vi "Motors 2.vi"(1 "Cluster":T1, 2 "Motors Visa Ref":refnum<visa-resource-name>="COM7") -> ()   [LabVIEW 2010]
panel:
  in  "Steps to deactivate hard limit after finding datums":dbl=500.0
  out "Loop i":i32
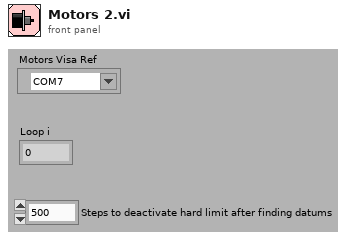
[diagram p1: front panel]
types:
  T1 = cluster{"Stop X?":refnum<vi>, "Stop Y?":refnum<vi>, "Stop Z?":refnum<vi>, "Stop Theta?":refnum<vi>, "Backlash?":refnum<vi>, "Backlash X":refnum<vi>, "Backlash Y":refnum<vi>, "Backlash Z":refnum<vi>, "Backlash Theta":refnum<vi>, "Manual IO?":refnum<vi>, "Manual Communication is Active\n(Close Before Ending Program)":refnum<vi>, "Reset Motors?":refnum<vi>, "Set Jogger?":refnum<vi>, "Normal":refnum<vi>, "Fast":refnum<vi>, "Jogger Axis":refnum<vi>, "Redefine Origin as Current Location?":refnum<vi>, "Save Current Motor Parameters?":refnum<vi>, "Find Datums Nearest Hard Limits?":refnum<vi>, "Saved Limits":refnum<vi>, "Use Datums Nearest Hard Limits to Reset Origin?":refnum<vi>, "X Go?":refnum<vi>, "Y Go?":refnum<vi>, "Z Go?":refnum<vi>, "Theta Go?":refnum<vi>, "Jog-Mode":refnum<vi>, "x+?":refnum<vi>, "x-?":refnum<vi>, "y+?":refnum<vi>, "y-?":refnum<vi>, "z+?":refnum<vi>, "z-?":refnum<vi>, "theta+?":refnum<vi>, "theta-?":refnum<vi>, "X Set Slew Speed?":refnum<vi>, "(mm/s)":refnum<vi>, "Y Set Slew Speed?":refnum<vi>, "(mm/s)":refnum<vi>, "Z Set Slew Speed?":refnum<vi>, "(mm/s)":refnum<vi>, "Theta Set Slew Speed?":refnum<vi>, "(degrees/s)":refnum<vi>, "Go To Saved Position?":refnum<vi>, "Defined Positions":refnum<vi>, "Need to Update Motor Parameters":refnum<vi>, "X Jogger Normal Speed":refnum<vi>, "X Jogger Fast Speed":refnum<vi>, "Y Jogger Normal Speed":refnum<vi>, "Y Jogger Fast Speed":refnum<vi>, "Z Jogger Normal Speed":refnum<vi>, "Z Jogger Fast Speed":refnum<vi>, "Theta Jogger Normal Speed":refnum<vi>, "Theta Jogger Fast Speed":refnum<vi>, "X Moving":refnum<vi>, "Y Moving":refnum<vi>, "Z Moving":refnum<vi>, "Theta Moving":refnum<vi>, "X Slew Speed (mm or degree/s)":refnum<vi>, "Y Slew Speed (mm or degree/s)":refnum<vi>, "Z Slew Speed (mm or degree/s)":refnum<vi>, "Theta Slew Speed (mm or degree/s)":refnum<vi>, "X-Axis (mm)":refnum<vi>, "Y-Axis (mm)":refnum<vi>, "Z-Axis (mm)":refnum<vi>, "Theta (deg)":refnum<vi>, "X Multiplier":refnum<vi>, "Y Multiplier":refnum<vi>, "Z Multiplier":refnum<vi>, "Theta Multiplier":refnum<vi>, "Motors Online":refnum<vi>, "Motors Status":refnum<vi>, "Status X":refnum<vi>, "Status Y":refnum<vi>, "Status Z":refnum<vi>, "Status Theta":refnum<vi>, "Motors error":refnum<vi>, "QUIT":refnum<vi>, "EMERGENCY":refnum<vi>, "X Go To":refnum<vi>, "Y Go To":refnum<vi>, "Z Go To":refnum<vi>, "Theta Go To":refnum<vi>, "Delta X (mm)":refnum<vi>, "Delta Y (mm)":refnum<vi>, "Delta Z (mm)":refnum<vi>, "Delta Theta (deg)":refnum<vi>, "X Speed (mm/s)":refnum<vi>, "Y Speed (mm/s)":refnum<vi>, "Z Speed (mm/s)":refnum<vi>, "Theta Speed (deg/s)":refnum<vi>, "x+":refnum<vi>, "x-":refnum<vi>, "y+":refnum<vi>, "y-":refnum<vi>, "z+":refnum<vi>, "z-":refnum<vi>, "theta+":refnum<vi>, "theta-":refnum<vi>, "Saved Positions":refnum<vi>}
  T2 = cluster{"X Set Slew Speed?":refnum<vi>, "(mm/s)":refnum<vi>, "Y Set Slew Speed?":refnum<vi>, "(mm/s)":refnum<vi>, "Z Set Slew Speed?":refnum<vi>, "(mm/s)":refnum<vi>, "Theta Set Slew Speed?":refnum<vi>, "(degrees/s)":refnum<vi>, "Need to Update Motor Parameters":refnum<vi>, "X Multiplier":refnum<vi>, "Y Multiplier":refnum<vi>, "Z Multiplier":refnum<vi>, "Theta Multiplier":refnum<vi>}
  T3 = cluster{"Jog-Mode":refnum<vi>, "y+?":refnum<vi>, "y-?":refnum<vi>, "Y Moving":refnum<vi>, "Delta Y (mm)":refnum<vi>, "Y Multiplier":refnum<vi>, "y+":refnum<vi>, "y-":refnum<vi>, "Y-Axis (mm)":refnum<vi>, "Status Y":refnum<vi>, "Y Speed (mm/s)":refnum<vi>}
  T4 = cluster{"Jog-Mode":refnum<vi>, "z+?":refnum<vi>, "z-?":refnum<vi>, "Z Speed (mm/s)":refnum<vi>, "Delta Z (mm)":refnum<vi>, "Z Multiplier":refnum<vi>, "Z-Axis (mm)":refnum<vi>, "Status Z":refnum<vi>, "z+":refnum<vi>, "z-":refnum<vi>, "Z Moving":refnum<vi>}
  T5 = cluster{"Jog-Mode":refnum<vi>, "theta+?":refnum<vi>, "theta-?":refnum<vi>, "Theta Speed (deg/s)":refnum<vi>, "Delta Theta (deg)":refnum<vi>, "Theta Multiplier":refnum<vi>, "Theta (deg)":refnum<vi>, "Status Theta":refnum<vi>, "theta+":refnum<vi>, "theta-":refnum<vi>, "Theta Moving":refnum<vi>}
  T6 = cluster{"Stop X?":refnum<vi>, "Stop Y?":refnum<vi>, "Stop Z?":refnum<vi>, "Stop Theta?":refnum<vi>}
  T7 = cluster{"Backlash?":refnum<vi>, "Backlash X":refnum<vi>, "Backlash Y":refnum<vi>, "Backlash Z":refnum<vi>, "Backlash Theta":refnum<vi>}
  T8 = cluster{"EMERGENCY":refnum<vi>, "Manual IO?":refnum<vi>, "Manual Communication is Active\n(Close Before Ending Program)":refnum<vi>, "Reset Motors?":refnum<vi>}
  T9 = cluster{"Redefine Origin as Current Location?":refnum<vi>, "Save Current Motor Parameters?":refnum<vi>}
  T10 = cluster{"Set Jogger?":refnum<vi>, "Normal":refnum<vi>, "Fast":refnum<vi>, "Jogger Axis":refnum<vi>, "X Multiplier":refnum<vi>, "Y Multiplier":refnum<vi>, "Z Multiplier":refnum<vi>, "Theta Multiplier":refnum<vi>, "Need to Update Motor Parameters":refnum<vi>}
  T11 = cluster{"Find Datums Nearest Hard Limits?":refnum<vi>, "X Multiplier":refnum<vi>, "Y Multiplier":refnum<vi>, "Z Multiplier":refnum<vi>, "Theta Multiplier":refnum<vi>, "X-Axis (mm)":refnum<vi>, "Y-Axis (mm)":refnum<vi>, "Z-Axis (mm)":refnum<vi>, "Theta (deg)":refnum<vi>, "Status X":refnum<vi>, "Status Y":refnum<vi>, "Status Z":refnum<vi>, "Status Theta":refnum<vi>, "X Moving":refnum<vi>, "Y Moving":refnum<vi>, "Z Moving":refnum<vi>, "Theta Moving":refnum<vi>, "Saved Limits":refnum<vi>}
  T12 = cluster{"Use Datums Nearest Hard Limits to Reset Origin?":refnum<vi>, "X Multiplier":refnum<vi>, "Y Multiplier":refnum<vi>, "Z Multiplier":refnum<vi>, "Theta Multiplier":refnum<vi>, "X-Axis (mm)":refnum<vi>, "Y-Axis (mm)":refnum<vi>, "Z-Axis (mm)":refnum<vi>, "Theta (deg)":refnum<vi>, "Status X":refnum<vi>, "Status Y":refnum<vi>, "Status Z":refnum<vi>, "Status Theta":refnum<vi>}
  T13 = cluster{"X Go?":refnum<vi>, "X Multiplier":refnum<vi>, "X Go To":refnum<vi>, "Y Go?":refnum<vi>, "Y Multiplier":refnum<vi>, "Y Go To":refnum<vi>, "Z Go?":refnum<vi>, "Z Multiplier":refnum<vi>, "Z Go To":refnum<vi>, "Theta Go?":refnum<vi>, "Theta Multiplier":refnum<vi>, "Theta Go To":refnum<vi>}
  T14 = cluster{"Jog-Mode":refnum<vi>, "x+?":refnum<vi>, "x-?":refnum<vi>, "X Moving":refnum<vi>, "X Multiplier":refnum<vi>, "Delta X (mm)":refnum<vi>, "X Speed (mm/s)":refnum<vi>, "x+":refnum<vi>, "x-":refnum<vi>, "X-Axis (mm)":refnum<vi>, "Status X":refnum<vi>}
  T15 = cluster{"Go To Saved Position?":refnum<vi>, "Defined Positions":refnum<vi>, "X Multiplier":refnum<vi>, "Y Multiplier":refnum<vi>, "Z Multiplier":refnum<vi>, "Theta Multiplier":refnum<vi>, void}
  T16 = cluster{"Status X":refnum<vi>, "X-Axis (mm)":refnum<vi>, "X Multiplier":refnum<vi>, "X Moving":refnum<vi>, "Status Y":refnum<vi>, "Y-Axis (mm)":refnum<vi>, "Y Multiplier":refnum<vi>, "Y Moving":refnum<vi>, "Status Z":refnum<vi>, "Z-Axis (mm)":refnum<vi>, "Z Multiplier":refnum<vi>, "Z Moving":refnum<vi>, "Status Theta":refnum<vi>, "Theta (deg)":refnum<vi>, "Theta Multiplier":refnum<vi>, "Theta Moving":refnum<vi>}
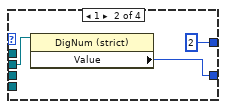
[diagram p3: hidden frame]
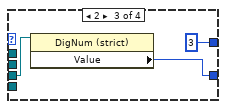
[diagram p4: hidden frame]
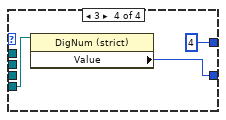
[diagram p5: hidden frame]
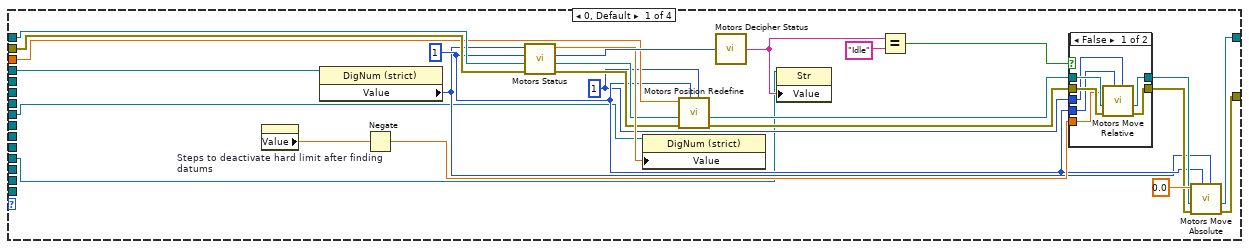
[diagram p15: hidden frame]
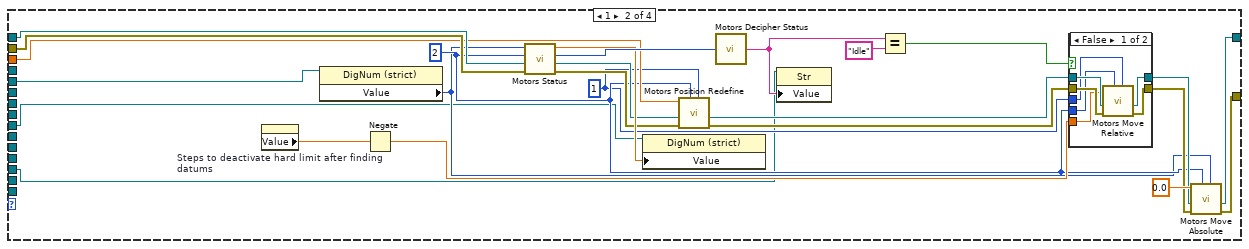
[diagram p17: hidden frame]
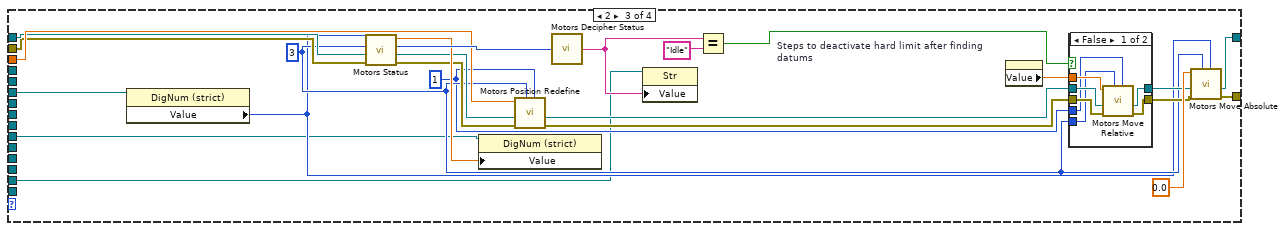
[diagram p19: hidden frame]
diagram:
  n1 = Unbundle("Cluster") -> ("Stop X?"=w101:refnum<vi>, "Stop Y?"=w100:refnum<vi>, "Stop Z?"=w99:refnum<vi>, "Stop Theta?"=w98:refnum<vi>, "Backlash?"=w97:refnum<vi>, "Backlash X"=w96:refnum<vi>, "Backlash Y"=w95:refnum<vi>, "Backlash Z"=w94:refnum<vi>, "Backlash Theta"=w93:refnum<vi>, "Manual IO?"=w91:refnum<vi>, "Manual Communication is Active\n(Close Before Ending Program)"=w90:refnum<vi>, "Reset Motors?"=w89:refnum<vi>, "Set Jogger?"=w85:refnum<vi>, "Normal"=w84:refnum<vi>, "Fast"=w83:refnum<vi>, "Jogger Axis"=w82:refnum<vi>, "Redefine Origin as Current Location?"=w80:refnum<vi>, "Save Current Motor Parameters?"=w79:refnum<vi>, "Find Datums Nearest Hard Limits?"=w77:refnum<vi>, "Saved Limits"=w71:refnum<vi>, "Use Datums Nearest Hard Limits to Reset Origin?"=w72:refnum<vi>, "X Go?"=w69:refnum<vi>, "Y Go?"=w67:refnum<vi>, "Z Go?"=w65:refnum<vi>, "Theta Go?"=w63:refnum<vi>, "Jog-Mode"=w41:refnum<vi>, "x+?"=w60:refnum<vi>, "x-?"=w59:refnum<vi>, "y+?"=w53:refnum<vi>, "y-?"=w52:refnum<vi>, "z+?"=w47:refnum<vi>, "z-?"=w46:refnum<vi>, "theta+?"=w40:refnum<vi>, "theta-?"=w39:refnum<vi>, "X Set Slew Speed?"=w31:refnum<vi>, "(mm/s)"=w30:refnum<vi>, "Y Set Slew Speed?"=w29:refnum<vi>, "(mm/s)"=w28:refnum<vi>, "Z Set Slew Speed?"=w27:refnum<vi>, "(mm/s)"=w26:refnum<vi>, "Theta Set Slew Speed?"=w25:refnum<vi>, "(degrees/s)"=w24:refnum<vi>, "Go To Saved Position?"=w8:refnum<vi>, "Defined Positions"=w7:refnum<vi>, "Need to Update Motor Parameters"=w23:refnum<vi>, "X Moving"=w13:refnum<vi>, "Y Moving"=w12:refnum<vi>, "Z Moving"=w11:refnum<vi>, "Theta Moving"=w10:refnum<vi>, "X-Axis (mm)"=w17:refnum<vi>, "Y-Axis (mm)"=w16:refnum<vi>, "Z-Axis (mm)"=w15:refnum<vi>, "Theta (deg)"=w14:refnum<vi>, "X Multiplier"=w6:refnum<vi>, "Y Multiplier"=w4:refnum<vi>, "Z Multiplier"=w3:refnum<vi>, "Theta Multiplier"=w5:refnum<vi>, "Motors Online"=w73:refnum<vi>, "Motors Status"=w76:refnum<vi>, "Status X"=w21:refnum<vi>, "Status Y"=w20:refnum<vi>, "Status Z"=w19:refnum<vi>, "Status Theta"=w18:refnum<vi>, "Motors error"=w74:refnum<vi>, "QUIT"=w105:refnum<vi>, "EMERGENCY"=w88:refnum<vi>, "X Go To"=w68:refnum<vi>, "Y Go To"=w66:refnum<vi>, "Z Go To"=w64:refnum<vi>, "Theta Go To"=w62:refnum<vi>, "Delta X (mm)"=w58:refnum<vi>, "Delta Y (mm)"=w51:refnum<vi>, "Delta Z (mm)"=w44:refnum<vi>, "Delta Theta (deg)"=w37:refnum<vi>, "X Speed (mm/s)"=w57:refnum<vi>, "Y Speed (mm/s)"=w48:refnum<vi>, "Z Speed (mm/s)"=w45:refnum<vi>, "Theta Speed (deg/s)"=w38:refnum<vi>, "x+"=w56:refnum<vi>, "x-"=w55:refnum<vi>, "y+"=w50:refnum<vi>, "y-"=w49:refnum<vi>, "z+"=w43:refnum<vi>, "z-"=w42:refnum<vi>, "theta+"=w36:refnum<vi>, "theta-"=w35:refnum<vi>)  [unwired: 13 out]
  n2 = Bundle("X Set Slew Speed?"=w31, "(mm/s)"=w30, "Y Set Slew Speed?"=w29, "(mm/s)"=w28, "Z Set Slew Speed?"=w27, "(mm/s)"=w26, "Theta Set Slew Speed?"=w25, "(degrees/s)"=w24, "Need to Update Motor Parameters"=w23, "X Multiplier"=w6, "Y Multiplier"=w4, "Z Multiplier"=w3, "Theta Multiplier"=w5) -> (w22:T2)  [unwired: 1 in]
  n3 = Bundle("Jog-Mode"=w41, "y+?"=w53, "y-?"=w52, "Y Moving"=w12, "Delta Y (mm)"=w51, "Y Multiplier"=w4, "y+"=w50, "y-"=w49, "Y-Axis (mm)"=w16, "Status Y"=w20, "Y Speed (mm/s)"=w48) -> (w34:T3)  [unwired: 1 in]
  n4 = Bundle("Jog-Mode"=w41, "z+?"=w47, "z-?"=w46, "Z Speed (mm/s)"=w45, "Delta Z (mm)"=w44, "Z Multiplier"=w3, "Z-Axis (mm)"=w15, "Status Z"=w19, "z+"=w43, "z-"=w42, "Z Moving"=w11) -> (w33:T4)  [unwired: 1 in]
  n5 = Bundle("Jog-Mode"=w41, "theta+?"=w40, "theta-?"=w39, "Theta Speed (deg/s)"=w38, "Delta Theta (deg)"=w37, "Theta Multiplier"=w5, "Theta (deg)"=w14, "Status Theta"=w18, "theta+"=w36, "theta-"=w35, "Theta Moving"=w10) -> (w32:T5)  [unwired: 1 in]
  n6 = Bundle("Stop X?"=w101, "Stop Y?"=w100, "Stop Z?"=w99, "Stop Theta?"=w98) -> (w87:T6)  [unwired: 1 in]
  n7 = Bundle("Backlash?"=w97, "Backlash X"=w96, "Backlash Y"=w95, "Backlash Z"=w94, "Backlash Theta"=w93) -> (w92:T7)  [unwired: 1 in]
  n8 = Bundle("EMERGENCY"=w88, "Manual IO?"=w91, "Manual Communication is Active\n(Close Before Ending Program)"=w90, "Reset Motors?"=w89) -> (w86:T8)  [unwired: 1 in]
  n9 = Bundle("Redefine Origin as Current Location?"=w80, "Save Current Motor Parameters?"=w79) -> (w78:T9)  [unwired: 1 in]
  n10 = Bundle("Set Jogger?"=w85, "Normal"=w84, "Fast"=w83, "Jogger Axis"=w82, "X Multiplier"=w6, "Y Multiplier"=w4, "Z Multiplier"=w3, "Theta Multiplier"=w5, "Need to Update Motor Parameters"=w23) -> (w81:T10)  [unwired: 1 in]
  n11 = Bundle("Find Datums Nearest Hard Limits?"=w77, "X Multiplier"=w6, "Y Multiplier"=w4, "Z Multiplier"=w3, "Theta Multiplier"=w5, "X-Axis (mm)"=w17, "Y-Axis (mm)"=w16, "Z-Axis (mm)"=w15, "Theta (deg)"=w14, "Status X"=w21, "Status Y"=w20, "Status Z"=w19, "Status Theta"=w18, "X Moving"=w13, "Y Moving"=w12, "Z Moving"=w11, "Theta Moving"=w10, "Saved Limits"=w71) -> (w75:T11)  [unwired: 1 in]
  n12 = Bundle("Use Datums Nearest Hard Limits to Reset Origin?"=w72, "X Multiplier"=w6, "Y Multiplier"=w4, "Z Multiplier"=w3, "Theta Multiplier"=w5, "X-Axis (mm)"=w17, "Y-Axis (mm)"=w16, "Z-Axis (mm)"=w15, "Theta (deg)"=w14, "Status X"=w21, "Status Y"=w20, "Status Z"=w19, "Status Theta"=w18) -> (w70:T12)  [unwired: 1 in]
  n13 = Bundle("X Go?"=w69, "X Multiplier"=w6, "X Go To"=w68, "Y Go?"=w67, "Y Multiplier"=w4, "Y Go To"=w66, "Z Go?"=w65, "Z Multiplier"=w3, "Z Go To"=w64, "Theta Go?"=w63, "Theta Multiplier"=w5, "Theta Go To"=w62) -> (w61:T13)  [unwired: 1 in]
  n14 = Bundle("Jog-Mode"=w41, "x+?"=w60, "x-?"=w59, "X Moving"=w13, "X Multiplier"=w6, "Delta X (mm)"=w58, "X Speed (mm/s)"=w57, "x+"=w56, "x-"=w55, "X-Axis (mm)"=w17, "Status X"=w21) -> (w54:T14)  [unwired: 1 in]
  n15 = property on="Property Node" class="Str"(reference=w76, "Value"="Opening Communications") -> (reference out=w104:refnum<vi>)  [unwired: 1 in, 1 out]
  n16 = call "Motors Open.vi"("VISA in"="Motors Visa Ref") -> ("error out"=w109:errorcluster, "VISA out"=w106:refnum<visa-resource-name>)  [unwired: 1 in]
  n17 = property on="Property Node" class="Bool (strict)"(reference=w23, "Value"=TRUE) -> ()  [unwired: 1 in, 2 out]
  n18 = call <vilib>:"Simple Error Handler.vi"("error in (no error)"=w109) -> ("error?"=w108:bool, "error out"=w110:errorcluster)  [unwired: 4 in, 3 out]
  n19 = property on="Property Node" class="Clust (strict)"(reference=w74, "Value"=w110) -> ()  [unwired: 1 in, 2 out]
  n20 = Bundle("Go To Saved Position?"=w8, "Defined Positions"=w7, "X Multiplier"=w6, "Y Multiplier"=w4, "Z Multiplier"=w3, "Theta Multiplier"=w5) -> (w2:T15)  [unwired: 2 in]
  n21 = Bundle("Status X"=w21, "X-Axis (mm)"=w17, "X Multiplier"=w6, "X Moving"=w13, "Status Y"=w20, "Y-Axis (mm)"=w16, "Y Multiplier"=w4, "Y Moving"=w12, "Status Z"=w19, "Z-Axis (mm)"=w15, "Z Multiplier"=w3, "Z Moving"=w11, "Status Theta"=w18, "Theta (deg)"=w14, "Theta Multiplier"=w5, "Theta Moving"=w10) -> (w9:T16)  [unwired: 1 in]
  n22 = Not(x=w108) -> (.not. x?=w107:bool)
  n23 = case shown="True" w107 {
    tunnel: w104 -> [_ w131]
    tunnel: w106 -> [_ w130]
    tunnel: w74 -> [_ w129]
    tunnel: w105 -> [_ w128]
    tunnel: w92 -> [_ w126]
    tunnel: w87 -> [_ w125]
    tunnel: w86 -> [_ w124]
    tunnel: w81 -> [_ w123]
    tunnel: w78 -> [_ w122]
    tunnel: w75 -> [_ w121]
    tunnel: w70 -> [_ w120]
    tunnel: w61 -> [_ w119]
    tunnel: w54 -> [_ w118]
    tunnel: w34 -> [_ w117]
    tunnel: w33 -> [_ w116]
    tunnel: w32 -> [_ w115]
    tunnel: w22 -> [_ w114]
    tunnel: w9 -> [_ w113]
    tunnel: w2 -> [_ w112]
    frame False {
    }
    frame True {
      n24 = property on="Property Node" class="Str"(reference=w131, "Value"="Running") -> (reference out=w127:refnum<vi>)  [unwired: 1 in, 1 out]
      n25 = while {
        shift-right: _ -> [_]
        shift-left: w130 -> [w324]
        tunnel: w129 -> [w421]
        tunnel: w128 -> [w368]
        tunnel: w127 -> [w365]
        tunnel: w126 -> [w313]
        tunnel: w125 -> [w325]
        tunnel: w124 -> [w302]
        tunnel: w123 -> [w284]
        tunnel: w122 -> [w283]
        tunnel: w121 -> [w278]
        tunnel: w120 -> [w259]
        tunnel: w119 -> [w245]
        tunnel: w118 -> [w232]
        tunnel: w117 -> [w218]
        tunnel: w116 -> [w203]
        tunnel: w115 -> [w190]
        tunnel: w114 -> [w176]
        tunnel: w113 -> [w154]
        tunnel: w112 -> [w137]
        i -> [w369]
        stop <- w422 stop-if-true
        # "This loop contains all of the code that has to communicate directly with the manipulator motor controllers.  They are arranged linearly to ensure multiple serial I/O's are never attempted simultaneously.  Note that this loop executes very slowly (each serial I/O takes about 1/20 sec)."
        n26 = Unbundle(w325) -> ("Stop X?"=w340:refnum<vi>, "Stop Y?"=w341:refnum<vi>, "Stop Z?"=w342:refnum<vi>, "Stop Theta?"=w343:refnum<vi>)
        n27 = property on="Property Node" class="Bool (strict)"(reference=w340) -> (reference out=w339:refnum<vi>, "Value"=w332:bool)  [unwired: 1 in, 1 out]
        n28 = property on="Property Node" class="Clust (strict)"(reference=w421) -> ("Value"=w323:errorcluster)  [unwired: 1 in, 2 out]
        n29 = case shown="True" w332 {
          tunnel: w323 -> [w528 w536]
          tunnel: w324 -> [w529 w535]
          tunnel: [w529 w533] -> w331
          tunnel: [w528 w532] -> w330
          tunnel: w339 -> [_ w530]
          frame False {
          }
          frame True {
            n30 = property on="Property Node" class="Bool (strict)"(reference=w530, "Value"=FALSE) -> ()  [unwired: 1 in, 2 out]
            n31 = call "Motors Stop.vi"("error in"=w536, "Axis"=1, "VISA in"=w535) -> ("error out"=w532:errorcluster, "VISA out"=w533:refnum<visa-resource-name>)
          }
        }
        n32 = property on="Property Node" class="Bool (strict)"(reference=w341) -> (reference out=w338:refnum<vi>, "Value"=w333:bool)  [unwired: 1 in, 1 out]
        n33 = case shown="True" w333 {
          tunnel: w330 -> [w519 w527]
          tunnel: w331 -> [w520 w526]
          tunnel: [w520 w524] -> w329
          tunnel: [w519 w523] -> w328
          tunnel: w338 -> [_ w521]
          frame False {
          }
          frame True {
            n34 = property on="Property Node" class="Bool (strict)"(reference=w521, "Value"=FALSE) -> ()  [unwired: 1 in, 2 out]
            n35 = call "Motors Stop.vi"("error in"=w527, "Axis"=2, "VISA in"=w526) -> ("error out"=w523:errorcluster, "VISA out"=w524:refnum<visa-resource-name>)
          }
        }
        n36 = property on="Property Node" class="Bool (strict)"(reference=w342) -> (reference out=w337:refnum<vi>, "Value"=w334:bool)  [unwired: 1 in, 1 out]
        n37 = case shown="True" w334 {
          tunnel: w328 -> [w510 w518]
          tunnel: w329 -> [w511 w517]
          tunnel: [w511 w515] -> w327
          tunnel: [w510 w514] -> w326
          tunnel: w337 -> [_ w512]
          frame False {
          }
          frame True {
            n38 = property on="Property Node" class="Bool (strict)"(reference=w512, "Value"=FALSE) -> ()  [unwired: 1 in, 2 out]
            n39 = call "Motors Stop.vi"("error in"=w518, "Axis"=3, "VISA in"=w517) -> ("error out"=w514:errorcluster, "VISA out"=w515:refnum<visa-resource-name>)
          }
        }
        n40 = property on="Property Node" class="Bool (strict)"(reference=w343) -> (reference out=w336:refnum<vi>, "Value"=w335:bool)  [unwired: 1 in, 1 out]
        n41 = case shown="True" w335 {
          tunnel: w326 -> [w501 w509]
          tunnel: w327 -> [w502 w508]
          tunnel: [w502 w506] -> w314
          tunnel: [w501 w505] -> w315
          tunnel: w336 -> [_ w503]
          frame False {
          }
          frame True {
            n42 = property on="Property Node" class="Bool (strict)"(reference=w503, "Value"=FALSE) -> ()  [unwired: 1 in, 2 out]
            n43 = call "Motors Stop.vi"("error in"=w509, "Axis"=4, "VISA in"=w508) -> ("error out"=w505:errorcluster, "VISA out"=w506:refnum<visa-resource-name>)
          }
        }
        n44 = Unbundle(w313) -> ("Backlash?"=w320:refnum<vi>, "Backlash X"=w316:refnum<vi>, "Backlash Y"=w317:refnum<vi>, "Backlash Z"=w318:refnum<vi>, "Backlash Theta"=w319:refnum<vi>)
        n45 = property on="Property Node" class="Bool (strict)"(reference=w320) -> (reference out=w322:refnum<vi>, "Value"=w321:bool)  [unwired: 1 in, 1 out]
        n46 = case shown="True" w321 {
          tunnel: [w486 w500] -> w301
          tunnel: w316 -> [_ w499]
          tunnel: w317 -> [_ w497]
          tunnel: w318 -> [_ w495]
          tunnel: w319 -> [_ w493]
          tunnel: w322 -> [_ w490]
          tunnel: w314 -> [w486 w489]
          tunnel: w315 -> [w485 w488]
          tunnel: [w485 w487] -> w300
          frame False {
          }
          frame True {
            n47 = property on="Property Node" class="Bool (strict)"(reference=w490, "Value"=FALSE) -> ()  [unwired: 1 in, 2 out]
            n48 = property on="Property Node" class="DigNum (strict)"(reference=w499) -> ("Value"=w498:u32)  [unwired: 1 in, 2 out]
            n49 = property on="Property Node" class="DigNum (strict)"(reference=w497) -> ("Value"=w496:u32)  [unwired: 1 in, 2 out]
            n50 = property on="Property Node" class="DigNum (strict)"(reference=w495) -> ("Value"=w494:u32)  [unwired: 1 in, 2 out]
            n51 = property on="Property Node" class="DigNum (strict)"(reference=w493) -> ("Value"=w492:u32)  [unwired: 1 in, 2 out]
            n52 = call "Motors Backlash.vi"("X"=w498, "Y"=w496, "VISA in"=w489, "error in"=w488, "Z"=w494, "Theta"=w492) -> ("VISA out"=w500:refnum<visa-resource-name>, "error out"=w487:errorcluster)  [unwired: 2 in]
          }
        }
        n53 = Unbundle(w302) -> ("EMERGENCY"=w305:refnum<vi>, "Manual IO?"=w308:refnum<vi>, "Manual Communication is Active\n(Close Before Ending Program)"=w306:refnum<vi>, "Reset Motors?"=w310:refnum<vi>)
        n54 = property on="Property Node" class="Bool (strict)"(reference=w308) -> (reference out=w309:refnum<vi>, "Value"=w307:bool)  [unwired: 1 in, 1 out]
        n55 = case shown="True" w307 {
          tunnel: [w458 w471] -> w304
          tunnel: [w459 w461] -> w303
          tunnel: w305 -> [_ w468]
          tunnel: w306 -> [_ w467]
          tunnel: w309 -> [_ w463]
          tunnel: w301 -> [w459 w462]
          tunnel: w300 -> [w458 w460]
          frame False {
          }
          frame True {
            n56 = property on="Property Node" class="Bool (strict)"(reference=w463, "Value"=FALSE) -> ()  [unwired: 1 in, 2 out]
            n57 = flat-sequence {
              tunnel: w467 -> [w473]
              tunnel: [w472] -> w465
              tunnel: [w480] -> w470
              tunnel: [w479] -> w469
              tunnel: w468 -> [w478]
              tunnel: [w477] -> w466
              tunnel: w465 -> [w477]
              tunnel: w462 -> [w476]
              tunnel: w460 -> [w475]
              tunnel: [w483] -> w461
              tunnel: [w484] -> w471
              tunnel: w470 -> [w484]
              tunnel: w469 -> [w483]
              tunnel: w466 -> [w481]
              frame #0 {
                n58 = property on="Property Node" class="Bool (strict)"(reference=w473, "Value"=TRUE ("Manual Communication is Active\n(Close Before Ending Program) 2")) -> (reference out=w472:refnum<vi>)  [unwired: 1 in, 1 out]
              }
              frame #1 {
                n59 = call "Motors Manual IO.vi"("error in"=w475, "Emergency Stop Reference"=w478, "VISA in"=w476) -> ("error out"=w480:errorcluster, "VISA out"=w479:refnum<visa-resource-name>)
              }
              frame #2 {
                n60 = property on="Property Node" class="Bool (strict)"(reference=w481, "Value"=FALSE ("Manual Communication is Active\n(Close Before Ending Program)")) -> ()  [unwired: 1 in, 2 out]
              }
            }
          }
        }
        n61 = Unbundle(w284) -> ("Set Jogger?"=w287:refnum<vi>, "Normal"=w289:refnum<vi>, "Fast"=w290:refnum<vi>, "Jogger Axis"=w293:refnum<vi>, "X Multiplier"=w295:refnum<vi>, "Y Multiplier"=w296:refnum<vi>, "Z Multiplier"=w297:refnum<vi>, "Theta Multiplier"=w298:refnum<vi>, "Need to Update Motor Parameters"=w299:refnum<vi>)
        n62 = property on="Property Node" class="Ring (strict)"(reference=w293) -> ("Value"=w294:u16)  [unwired: 1 in, 2 out]
        n63 = property on="Property Node" class="Bool (strict)"(reference=w310) -> (reference out=w312:refnum<vi>, "Value"=w311:bool)  [unwired: 1 in, 1 out]
        n64 = case shown="0, Default" w294 {
          tunnel: [u32 1 u32 2 u32 3 u32 4] -> _
          tunnel: [w424 w427 w430 w433] -> w292
          tunnel: w295 -> [w423 _ _ _]
          tunnel: w296 -> [_ w426 _ _]
          tunnel: w298 -> [_ _ _ w432]
          tunnel: w297 -> [_ _ w429 _]
          frame 0, Default {
            n65 = property on="Property Node" class="DigNum (strict)"(reference=w423) -> ("Value"=w424:u32)  [unwired: 1 in, 2 out]
          }
          frame 1 {
            n66 = property on="Property Node" class="DigNum (strict)"(reference=w426) -> ("Value"=w427:u32)  [unwired: 1 in, 2 out]
          }
          frame 2 {
            n67 = property on="Property Node" class="DigNum (strict)"(reference=w429) -> ("Value"=w430:u32)  [unwired: 1 in, 2 out]
          }
          frame 3 {
            n68 = property on="Property Node" class="DigNum (strict)"(reference=w432) -> ("Value"=w433:u32)  [unwired: 1 in, 2 out]
          }
        }
        n69 = case shown="True" w311 {
          tunnel: [w450 w457] -> w285
          tunnel: [w451 w456] -> w286
          tunnel: w303 -> [w451 w455]
          tunnel: w304 -> [w450 w454]
          tunnel: w312 -> [_ w452]
          frame False {
          }
          frame True {
            n70 = property on="Property Node" class="Bool (strict)"(reference=w452, "Value"=FALSE) -> ()  [unwired: 1 in, 2 out]
            n71 = call "Motors Reset.vi"("error in"=w454, "VISA in"=w455) -> ("error out"=w457:errorcluster, "VISA out"=w456:refnum<visa-resource-name>)
          }
        }
        n72 = property on="Property Node" class="Bool (strict)"(reference=w287) -> (reference out=w291:refnum<vi>, "Value"=w288:bool)  [unwired: 1 in, 1 out]
        n73 = case shown="True" w288 {
          tunnel: [w436 w449] -> w280
          tunnel: [w435 w447] -> w281
          tunnel: w292 -> [_ w448]
          tunnel: w291 -> [_ w445]
          tunnel: w289 -> [_ w441]
          tunnel: w290 -> [_ w440]
          tunnel: w285 -> [w436 w439]
          tunnel: w286 -> [w435 w438]
          tunnel: w299 -> [_ w437]
          frame False {
          }
          frame True {
            n74 = property on="Property Node" class="Bool (strict)"(reference=w445, "Value"=FALSE ("Need to Update Motor Parameters")) -> ()  [unwired: 1 in, 2 out]
            n75 = property on="Property Node" class="Bool (strict)"(reference=w437, "Value"=TRUE) -> ()  [unwired: 1 in, 2 out]
            n76 = property on="Property Node" class="DigNum (strict)"(reference=w441) -> ("Value"=w444:dbl)  [unwired: 1 in, 2 out]
            n77 = property on="Property Node" class="DigNum (strict)"(reference=w440) -> ("Value"=w443:dbl)  [unwired: 1 in, 2 out]
            n78 = call "Motors Jogger Speed.vi"("Axis Multiplier"=w448, "error in"=w439, "VISA in"=w438, "Fast Speed (mm or degree/sec)"=w443, "Normal Speed (mm or degree/sec)"=w444) -> ("error out"=w449:errorcluster, "VISA out"=w447:refnum<visa-resource-name>)  [unwired: 5 in]
          }
        }
        n79 = Unbundle(w283) -> ("Redefine Origin as Current Location?"=w282:refnum<vi>, "Save Current Motor Parameters?"=w279:refnum<vi>)
        n80 = property on="Property Node" class="Bool (strict)"(reference=w279) -> (reference out=w357:refnum<vi>, "Value"=w356:bool)  [unwired: 1 in, 1 out]
        n81 = property on="Property Node" class="Bool (strict)"(reference=w282) -> (reference out=w355:refnum<vi>, "Value"=w367:bool)  [unwired: 1 in, 1 out]
        n82 = case shown="True" w367 {
          tunnel: w281 -> [w1662 w1669]
          tunnel: w280 -> [w1663 w1665]
          tunnel: [w1663 w1667] -> w358
          tunnel: [w1662 w1668] -> w420
          tunnel: w355 -> [_ w1664]
          frame False {
          }
          frame True {
            n83 = property on="Property Node" class="Bool (strict)"(reference=w1664, "Value"=FALSE) -> ()  [unwired: 1 in, 2 out]
            n84 = call "Motors Redefine Origin.vi"("error in"=w1665, "VISA in"=w1669) -> ("error out"=w1667:errorcluster, "VISA out"=w1668:refnum<visa-resource-name>)
          }
        }
        n85 = case shown="True" w356 {
          tunnel: w358 -> [w1655 w1661]
          tunnel: [w1655 w1660] -> w375
          tunnel: w420 -> [w1654 w1659]
          tunnel: [w1654 w1658] -> w374
          tunnel: w357 -> [_ w1657]
          frame False {
          }
          frame True {
            n86 = property on="Property Node" class="Bool (strict)"(reference=w1657, "Value"=FALSE) -> ()  [unwired: 1 in, 2 out]
            n87 = call "Motors Save.vi"("error in"=w1661, "VISA in"=w1659) -> ("error out"=w1660:errorcluster, "VISA out"=w1658:refnum<visa-resource-name>)
          }
        }
        n88 = property on="Property Node" class="Bool (strict)"(reference=w368) -> ("Value"=w422:bool)  [unwired: 1 in, 2 out]
        n89 = Unbundle(w278) -> ("Find Datums Nearest Hard Limits?"=w277:refnum<vi>, "X Multiplier"=w276:refnum<vi>, "Y Multiplier"=w275:refnum<vi>, "Z Multiplier"=w274:refnum<vi>, "Theta Multiplier"=w273:refnum<vi>, "X-Axis (mm)"=w272:refnum<vi>, "Y-Axis (mm)"=w271:refnum<vi>, "Z-Axis (mm)"=w270:refnum<vi>, "Theta (deg)"=w269:refnum<vi>, "Status X"=w268:refnum<vi>, "Status Y"=w267:refnum<vi>, "Status Z"=w266:refnum<vi>, "Status Theta"=w265:refnum<vi>, "X Moving"=w264:refnum<vi>, "Y Moving"=w263:refnum<vi>, "Z Moving"=w262:refnum<vi>, "Theta Moving"=w261:refnum<vi>, "Saved Limits"=w260:refnum<vi>)
        n90 = property on="Property Node" class="Bool (strict)"(reference=w277) -> (reference out=w360:refnum<vi>, "Value"=w366:bool)  [unwired: 1 in, 1 out]
        n91 = case shown="True" w366 {
          tunnel: w375 -> [w754 w785]
          tunnel: [w754 w783] -> w372
          tunnel: [w753 w784] -> w370
          tunnel: w374 -> [w753 w786]
          tunnel: w365 -> [w752 w778]
          tunnel: [w751 w775] -> w363
          tunnel: [w752 w774] -> w362
          tunnel: w360 -> [_ w773]
          tunnel: w276 -> [_ w771]
          tunnel: w275 -> [_ w770]
          tunnel: w274 -> [_ w769]
          tunnel: w273 -> [_ w768]
          tunnel: w272 -> [_ w767]
          tunnel: w271 -> [_ w766]
          tunnel: w270 -> [_ w765]
          tunnel: w269 -> [_ w764]
          tunnel: w268 -> [_ w763]
          tunnel: w267 -> [_ w762]
          tunnel: w266 -> [_ w761]
          tunnel: w265 -> [_ w760]
          tunnel: w264 -> [_ w759]
          tunnel: w263 -> [_ w758]
          tunnel: w262 -> [_ w757]
          tunnel: w261 -> [_ w756]
          tunnel: w260 -> [w751 w755]
          frame False {
          }
          frame True {
            n92 = property on="Property Node" class="Bool (strict)"(reference=w773, "Value"=FALSE) -> ()  [unwired: 1 in, 2 out]
            n93 = flat-sequence {
              tunnel: w785 -> [w791]
              tunnel: w786 -> [w792]
              tunnel: [w792] -> w782
              tunnel: [w791] -> w781
              tunnel: w778 -> [w788]
              tunnel: [w787] -> w776
              tunnel: w782 -> [w828]
              tunnel: w781 -> [w827]
              tunnel: [w823] -> w780
              tunnel: [w822] -> w779
              tunnel: [w812] -> w777
              tunnel: w776 -> [w812]
              tunnel: [w810] -> w775
              tunnel: w771 -> [w809]
              tunnel: w770 -> [w808]
              tunnel: w769 -> [w807]
              tunnel: w768 -> [w806]
              tunnel: w767 -> [w805]
              tunnel: w766 -> [w804]
              tunnel: w765 -> [w803]
              tunnel: w764 -> [w802]
              tunnel: w763 -> [w801]
              tunnel: w762 -> [w800]
              tunnel: w761 -> [w799]
              tunnel: w760 -> [w798]
              tunnel: w759 -> [w797]
              tunnel: w758 -> [w796]
              tunnel: w757 -> [w795]
              tunnel: w756 -> [w794]
              tunnel: w755 -> [w793]
              tunnel: [w938] -> w783
              tunnel: [w939] -> w784
              tunnel: w780 -> [w939]
              tunnel: w779 -> [w938]
              tunnel: w777 -> [w936]
              tunnel: [w935] -> w774
              frame #0 {
                n94 = call <vilib>:"Set Busy.vi"("disable click? (T)"=FALSE) -> ()  [unwired: 9 in, 2 out]
                n95 = property on="Property Node" class="Str"(reference=w788, "Value"="Finding Datums Nearest Hard Limits\nThis May Take a Few Minutes" ("Status")) -> (reference out=w787:refnum<vi>)  [unwired: 1 in, 1 out]
              }
              frame #1 {
                n96 = call "Motors Find Datums.vi"("error in"=w827, "VISA in"=w828) -> ("error out"=w824:errorcluster, "VISA out"=w825:refnum<visa-resource-name>)
                n97 = for {
                  N: 4 -> [_]
                  shift-right: [w848] -> w822
                  shift-left: w824 -> [w849]
                  shift-right: [w847] -> w823
                  shift-left: w825 -> [w850]
                  tunnel: [w846] -> w814 mode=indexing
                  tunnel: w809 -> [w844]
                  tunnel: w808 -> [w843]
                  tunnel: w807 -> [w842]
                  tunnel: w806 -> [w841]
                  tunnel: w805 -> [w840]
                  tunnel: w804 -> [w839]
                  tunnel: w803 -> [w838]
                  tunnel: w802 -> [w837]
                  tunnel: w801 -> [w836]
                  tunnel: w800 -> [w835]
                  tunnel: w799 -> [w834]
                  tunnel: w798 -> [w833]
                  tunnel: w797 -> [w832]
                  tunnel: w796 -> [w831]
                  tunnel: w795 -> [w830]
                  tunnel: w794 -> [w829]
                  i -> [w845]
                  n98 = case shown="0, Default" w845 {
                    tunnel: w849 -> [w863 w884 w905 w926]
                    tunnel: w850 -> [w864 w885 w906 w927]
                    tunnel: [w857 w878 w898 w919] -> w848
                    tunnel: [w858 w879 w899 w920] -> w847
                    tunnel: [w855 w876 w902 w923] -> w846
                    tunnel: w844 -> [w854 _ _ _]
                    tunnel: w843 -> [_ w875 _ _]
                    tunnel: w842 -> [_ _ w896 _]
                    tunnel: w841 -> [_ _ _ w917]
                    tunnel: w840 -> [w853 _ _ _]
                    tunnel: w839 -> [_ w874 _ _]
                    tunnel: w838 -> [_ _ w895 _]
                    tunnel: w837 -> [_ _ _ w916]
                    tunnel: w836 -> [w852 _ _ _]
                    tunnel: w835 -> [_ w873 _ _]
                    tunnel: w834 -> [_ _ w894 _]
                    tunnel: w833 -> [_ _ _ w915]
                    tunnel: w832 -> [w851 _ _ _]
                    tunnel: w831 -> [_ w872 _ _]
                    tunnel: w830 -> [_ _ w893 _]
                    tunnel: w829 -> [_ _ _ w914]
                    frame 0, Default {
                      w856 = 1 ("Axis")
                      n99 = property on="Property Node" class="DigNum (strict)"(reference=w854) -> ("Value"=w862:u32)  [unwired: 1 in, 2 out]
                      n100 = call "Motors Status.vi"("error in"=w863, "VISA in"=w864, "Axis"=w856, "Axis Multiplier"=w862) -> ("error out"=w859:errorcluster, "VISA out"=w860:refnum<visa-resource-name>, "OS"=w869:i32, "Actual Position (mm or deg)"=w861:dbl)  [unwired: 3 in]
                      n101 = property on="Property Node" class="DigNum (strict)"(reference=w853, "Value"=w861) -> ()  [unwired: 1 in, 2 out]
                      n102 = call "Motors Datum Position.vi"("error in"=w859, "VISA in"=w860, "Axis"=w856) -> ("error out"=w857:errorcluster, "VISA out"=w858:refnum<visa-resource-name>, "Datum Position (steps)"=w855:string)  [unwired: 5 in]
                      n103 = call "Motors Decipher Status.vi"("OS"=w869) -> ("Status"=w868:string)
                      n104 = property on="Property Node" class="Str"(reference=w852, "Value"=w868) -> ()  [unwired: 1 in, 2 out]
                      n105 = Equal?(x=w868, y="Idle") -> (x = y?=w866:bool)
                      n106 = case shown="False" w866 {
                        tunnel: [TRUE FALSE] -> w865
                        frame False {
                        }
                        frame True {
                        }
                      }
                      n107 = property on="Property Node" class="Bool (strict)"(reference=w851, "Value"=w865) -> ()  [unwired: 1 in, 2 out]
                    }
                    frame 1 {
                      w877 = 2 ("Axis")
                      n108 = property on="Property Node" class="DigNum (strict)"(reference=w875) -> ("Value"=w883:u32)  [unwired: 1 in, 2 out]
                      n109 = call "Motors Status.vi"("error in"=w884, "VISA in"=w885, "Axis"=w877, "Axis Multiplier"=w883) -> ("error out"=w880:errorcluster, "VISA out"=w881:refnum<visa-resource-name>, "OS"=w890:i32, "Actual Position (mm or deg)"=w882:dbl)  [unwired: 3 in]
                      n110 = property on="Property Node" class="DigNum (strict)"(reference=w874, "Value"=w882) -> ()  [unwired: 1 in, 2 out]
                      n111 = call "Motors Datum Position.vi"("error in"=w880, "VISA in"=w881, "Axis"=w877) -> ("error out"=w878:errorcluster, "VISA out"=w879:refnum<visa-resource-name>, "Datum Position (steps)"=w876:string)  [unwired: 5 in]
                      n112 = call "Motors Decipher Status.vi"("OS"=w890) -> ("Status"=w888:string)
                      n113 = property on="Property Node" class="Str"(reference=w873, "Value"=w888) -> ()  [unwired: 1 in, 2 out]
                      n114 = Equal?(x=w888, y="Idle") -> (x = y?=w887:bool)
                      n115 = case shown="False" w887 {
                        tunnel: [TRUE FALSE] -> w886
                        frame False {
                        }
                        frame True {
                        }
                      }
                      n116 = property on="Property Node" class="Bool (strict)"(reference=w872, "Value"=w886) -> ()  [unwired: 1 in, 2 out]
                    }
                    frame 2 {
                      w897 = 3 ("Axis")
                      n117 = property on="Property Node" class="DigNum (strict)"(reference=w896) -> ("Value"=w904:u32)  [unwired: 1 in, 2 out]
                      n118 = call "Motors Status.vi"("error in"=w905, "VISA in"=w906, "Axis"=w897, "Axis Multiplier"=w904) -> ("error out"=w900:errorcluster, "VISA out"=w901:refnum<visa-resource-name>, "OS"=w911:i32, "Actual Position (mm or deg)"=w903:dbl)  [unwired: 3 in]
                      n119 = property on="Property Node" class="DigNum (strict)"(reference=w895, "Value"=w903) -> ()  [unwired: 1 in, 2 out]
                      n120 = call "Motors Datum Position.vi"("error in"=w900, "VISA in"=w901, "Axis"=w897) -> ("error out"=w898:errorcluster, "VISA out"=w899:refnum<visa-resource-name>, "Datum Position (steps)"=w902:string)  [unwired: 5 in]
                      n121 = call "Motors Decipher Status.vi"("OS"=w911) -> ("Status"=w909:string)
                      n122 = property on="Property Node" class="Str"(reference=w894, "Value"=w909) -> ()  [unwired: 1 in, 2 out]
                      n123 = Equal?(x=w909, y="Idle") -> (x = y?=w908:bool)
                      n124 = case shown="False" w908 {
                        tunnel: [TRUE FALSE] -> w907
                        frame False {
                        }
                        frame True {
                        }
                      }
                      n125 = property on="Property Node" class="Bool (strict)"(reference=w893, "Value"=w907) -> ()  [unwired: 1 in, 2 out]
                    }
                    frame 3 {
                      w918 = 4 ("Axis")
                      n126 = property on="Property Node" class="DigNum (strict)"(reference=w917) -> ("Value"=w925:u32)  [unwired: 1 in, 2 out]
                      n127 = call "Motors Status.vi"("error in"=w926, "VISA in"=w927, "Axis"=w918, "Axis Multiplier"=w925) -> ("error out"=w921:errorcluster, "VISA out"=w922:refnum<visa-resource-name>, "OS"=w932:i32, "Actual Position (mm or deg)"=w924:dbl)  [unwired: 3 in]
                      n128 = property on="Property Node" class="DigNum (strict)"(reference=w916, "Value"=w924) -> ()  [unwired: 1 in, 2 out]
                      n129 = call "Motors Datum Position.vi"("error in"=w921, "VISA in"=w922, "Axis"=w918) -> ("error out"=w919:errorcluster, "VISA out"=w920:refnum<visa-resource-name>, "Datum Position (steps)"=w923:string)  [unwired: 5 in]
                      n130 = call "Motors Decipher Status.vi"("OS"=w932) -> ("Status"=w930:string)
                      n131 = property on="Property Node" class="Str"(reference=w915, "Value"=w930) -> ()  [unwired: 1 in, 2 out]
                      n132 = Equal?(x=w930, y="Idle") -> (x = y?=w929:bool)
                      n133 = case shown="True" w929 {
                        tunnel: [TRUE FALSE] -> w928
                        frame False {
                        }
                        frame True {
                        }
                      }
                      n134 = property on="Property Node" class="Bool (strict)"(reference=w914, "Value"=w928) -> ()  [unwired: 1 in, 2 out]
                    }
                  }
                }
                n135 = Build Array (concatenate)("Limits", w814) -> (w813:string[])
                n136 = Initialize Array("", 0 ("dimension size"), 0 ("dimension size")) -> (w820:string[][])
                n137 = Build Array (concatenate)(w813, w820) -> (w818:string[][])
                n138 = property on="Property Node" class="Path"(reference=w793) -> (reference out=w810:refnum<vi>, "Value"=w811:path)  [unwired: 1 in, 1 out]
                n139 = Transpose 2D Array(2D array=w818) -> (transposed array=w817:string[][])
                n140 = call "Motors Position Rewrite.vi"("file path"=w811, "Array of Positions"=w817) -> ()  [unwired: 9 in]
              }
              frame #2 {
                n141 = call <vilib>:"Unset Busy.vi"() -> ()  [unwired: 11 in, 1 out]
                n142 = property on="Property Node" class="Str"(reference=w936, "Value"="Running" ("Status")) -> (reference out=w935:refnum<vi>)  [unwired: 1 in, 1 out]
              }
            }
          }
        }
        n143 = Unbundle(w259) -> ("Use Datums Nearest Hard Limits to Reset Origin?"=w258:refnum<vi>, "X Multiplier"=w257:refnum<vi>, "Y Multiplier"=w256:refnum<vi>, "Z Multiplier"=w255:refnum<vi>, "Theta Multiplier"=w254:refnum<vi>, "X-Axis (mm)"=w253:refnum<vi>, "Y-Axis (mm)"=w252:refnum<vi>, "Z-Axis (mm)"=w251:refnum<vi>, "Theta (deg)"=w250:refnum<vi>, "Status X"=w249:refnum<vi>, "Status Y"=w248:refnum<vi>, "Status Z"=w247:refnum<vi>, "Status Theta"=w246:refnum<vi>)
        n144 = property on="Property Node" class="Bool (strict)"(reference=w258) -> (reference out=w359:refnum<vi>, "Value"=w364:bool)  [unwired: 1 in, 1 out]
        n145 = case shown="True" w364 {
          tunnel: [w539 w560] -> w373
          tunnel: w372 -> [w539 w562]
          tunnel: [w538 w559] -> w371
          tunnel: w370 -> [w538 w563]
          tunnel: w363 -> [_ w558]
          tunnel: w362 -> [w537 w554]
          tunnel: [w537 w555] -> _
          tunnel: w359 -> [_ w553]
          tunnel: w257 -> [_ w551]
          tunnel: w256 -> [_ w550]
          tunnel: w255 -> [_ w549]
          tunnel: w254 -> [_ w548]
          tunnel: w253 -> [_ w547]
          tunnel: w252 -> [_ w546]
          tunnel: w251 -> [_ w545]
          tunnel: w250 -> [_ w544]
          tunnel: w249 -> [_ w543]
          tunnel: w248 -> [_ w542]
          tunnel: w247 -> [_ w541]
          tunnel: w246 -> [_ w540]
          frame False {
          }
          frame True {
            n146 = property on="Property Node" class="Bool (strict)"(reference=w553, "Value"=FALSE) -> ()  [unwired: 1 in, 2 out]
            n147 = flat-sequence {
              tunnel: w562 -> [w567]
              tunnel: [w567] -> w561
              tunnel: w554 -> [w565]
              tunnel: [w564] -> w556
              tunnel: w563 -> [w591]
              tunnel: w561 -> [w592]
              tunnel: [w587] -> w560
              tunnel: [w586] -> w559
              tunnel: w558 -> [w582]
              tunnel: [w580] -> w557
              tunnel: w556 -> [w580]
              tunnel: w551 -> [w579]
              tunnel: w550 -> [w578]
              tunnel: w549 -> [w577]
              tunnel: w548 -> [w576]
              tunnel: w547 -> [w575]
              tunnel: w546 -> [w574]
              tunnel: w545 -> [w573]
              tunnel: w544 -> [w572]
              tunnel: w543 -> [w571]
              tunnel: w542 -> [w570]
              tunnel: w541 -> [w569]
              tunnel: w540 -> [w568]
              tunnel: w557 -> [w749]
              tunnel: [w748] -> w555
              frame #0 {
                n148 = call <vilib>:"Set Busy.vi"() -> ()  [unwired: 10 in, 2 out]
                n149 = property on="Property Node" class="Str"(reference=w565, "Value"="Finding Datums Nearest Hard Limits\nThis May Take a Few Minutes" ("Status")) -> (reference out=w564:refnum<vi>)  [unwired: 1 in, 1 out]
              }
              frame #1 {
                n150 = property on="Property Node" class="Path"(reference=w582) -> ("Value"=w581:path)  [unwired: 1 in, 2 out]
                n151 = call "Motors Find Datums.vi"("error in"=w592, "VISA in"=w591) -> ("error out"=w589:errorcluster, "VISA out"=w590:refnum<visa-resource-name>)
                n152 = call "Motors Position Load.vi"("error in"=w589, "file path"=w581) -> ("error out"=w588:errorcluster, "Positions"=w585:string[][])
                n153 = Delete From Array(array=w585, index (row)=0) -> (array with subset deleted=w583:string[][])  [unwired: 2 in, 1 out]
                n154 = for {
                  shift-right: [w611] -> w587
                  shift-left: w588 -> [w612]
                  shift-right: [w610] -> w586
                  shift-left: w590 -> [w613]
                  tunnel: w583 -> [w609] mode=indexing
                  tunnel: w579 -> [w604]
                  tunnel: w578 -> [w603]
                  tunnel: w577 -> [w602]
                  tunnel: w576 -> [w601]
                  tunnel: w575 -> [w600]
                  tunnel: w574 -> [w599]
                  tunnel: w573 -> [w598]
                  tunnel: w572 -> [w597]
                  tunnel: w571 -> [w596]
                  tunnel: w570 -> [w595]
                  tunnel: w569 -> [w594]
                  tunnel: w568 -> [w593]
                  i -> [w606]
                  n155 = Index Array(array=w609, index=0) -> (element=w608:string)
                  n156 = Fract/Exp String To Number(string=w608) -> (number=w607:dbl)  [unwired: 3 in, 1 out]
                  n157 = case shown="3" w606 {
                    tunnel: w612 -> [w633 w667 w697 w733]
                    tunnel: w613 -> [w634 w668 w698 w734]
                    tunnel: [w627 w660 w689 w726] -> w611
                    tunnel: [w628 w661 w690 w727] -> w610
                    tunnel: w607 -> [w629 w663 w700 w729]
                    tunnel: w604 -> [w616 _ _ _]
                    tunnel: w603 -> [_ w650 _ _]
                    tunnel: w602 -> [_ _ w684 _]
                    tunnel: w601 -> [_ _ _ w717]
                    tunnel: w600 -> [w615 _ _ _]
                    tunnel: w599 -> [_ w649 _ _]
                    tunnel: w598 -> [_ _ w683 _]
                    tunnel: w597 -> [_ _ _ w716]
                    tunnel: w596 -> [w614 _ _ _]
                    tunnel: w595 -> [_ w648 _ _]
                    tunnel: w594 -> [_ _ w682 _]
                    tunnel: w593 -> [_ _ _ w715]
                    frame 0, Default {
                      w617 = u32 1 ("Axis Multiplier")
                      w619 = 1 ("Axis")
                      n158 = property on="Steps to deactivate hard limit after finding datums" class="DigNum (strict)"() -> ("Value"=w625:dbl)  [unwired: 2 in, 2 out]
                      n159 = property on="Property Node" class="DigNum (strict)"(reference=w616) -> ("Value"=w618:u32)  [unwired: 1 in, 2 out]
                      n160 = Negate(x=w625) -> (-x=w620:dbl)
                      n161 = call "Motors Status.vi"("error in"=w633, "VISA in"=w634, "Axis"=w619, "Axis Multiplier"=w618) -> ("error out"=w630:errorcluster, "VISA out"=w631:refnum<visa-resource-name>, "OS"=w638:i32, "Actual Position (mm or deg)"=w632:dbl)  [unwired: 3 in]
                      n162 = property on="Property Node" class="DigNum (strict)"(reference=w615, "Value"=w632) -> ()  [unwired: 1 in, 2 out]
                      n163 = call "Motors Position Redefine.vi"("Axis Multiplier"=w617, "Axis"=w619, "error in"=w630, "VISA in"=w631, "Position (mm or deg)"=w629) -> ("error out"=w624:errorcluster, "VISA out"=w621:refnum<visa-resource-name>)  [unwired: 5 in]
                      n164 = call "Motors Decipher Status.vi"("OS"=w638) -> ("Status"=w637:string)
                      n165 = property on="Property Node" class="Str"(reference=w614, "Value"=w637) -> ()  [unwired: 1 in, 2 out]
                      n166 = Equal?(x=w637, y="Idle") -> (x = y?=w635:bool)
                      n167 = case shown="False" w635 {
                        tunnel: w624 -> [w645 w647]
                        tunnel: [w644 w647] -> w623
                        tunnel: w621 -> [w643 w646]
                        tunnel: [w642 w646] -> w622
                        tunnel: w620 -> [w641 _]
                        tunnel: w619 -> [w640 _]
                        tunnel: w617 -> [w639 _]
                        frame False {
                          n168 = call "Motors Move Relative.vi"("Axis Multiplier"=w639, "Axis"=w640, "error in"=w645, "VISA in"=w643, "Distance (mm)"=w641) -> ("error out"=w644:errorcluster, "VISA out"=w642:refnum<visa-resource-name>)  [unwired: 5 in]
                        }
                        frame True {
                        }
                      }
                      n169 = call "Motors Move Absolute.vi"("Axis Multiplier"=w618, "Axis"=w619, "error in"=w623, "VISA in"=w622, "Position (mm or degree)"=0.0) -> ("error out"=w627:errorcluster, "VISA out"=w628:refnum<visa-resource-name>)  [unwired: 5 in]
                    }
                    frame 1 {
                      w651 = u32 1 ("Axis Multiplier")
                      w653 = 2 ("Axis")
                      n170 = property on="Steps to deactivate hard limit after finding datums" class="DigNum (strict)"() -> ("Value"=w659:dbl)  [unwired: 2 in, 2 out]
                      n171 = property on="Property Node" class="DigNum (strict)"(reference=w650) -> ("Value"=w652:u32)  [unwired: 1 in, 2 out]
                      n172 = Negate(x=w659) -> (-x=w654:dbl)
                      n173 = call "Motors Status.vi"("error in"=w667, "VISA in"=w668, "Axis"=w653, "Axis Multiplier"=w652) -> ("error out"=w664:errorcluster, "VISA out"=w665:refnum<visa-resource-name>, "OS"=w672:i32, "Actual Position (mm or deg)"=w666:dbl)  [unwired: 3 in]
                      n174 = property on="Property Node" class="DigNum (strict)"(reference=w649, "Value"=w666) -> ()  [unwired: 1 in, 2 out]
                      n175 = call "Motors Position Redefine.vi"("Axis Multiplier"=w651, "Axis"=w653, "error in"=w664, "VISA in"=w665, "Position (mm or deg)"=w663) -> ("error out"=w657:errorcluster, "VISA out"=w658:refnum<visa-resource-name>)  [unwired: 5 in]
                      n176 = call "Motors Decipher Status.vi"("OS"=w672) -> ("Status"=w670:string)
                      n177 = property on="Property Node" class="Str"(reference=w648, "Value"=w670) -> ()  [unwired: 1 in, 2 out]
                      n178 = Equal?(x=w670, y="Idle") -> (x = y?=w669:bool)
                      n179 = case shown="False" w669 {
                        tunnel: w658 -> [w679 w680]
                        tunnel: w657 -> [w678 w681]
                        tunnel: [w677 w680] -> w656
                        tunnel: [w676 w681] -> w655
                        tunnel: w654 -> [w675 _]
                        tunnel: w653 -> [w674 _]
                        tunnel: w651 -> [w673 _]
                        frame False {
                          n180 = call "Motors Move Relative.vi"("Axis Multiplier"=w673, "Axis"=w674, "error in"=w678, "VISA in"=w679, "Distance (mm)"=w675) -> ("error out"=w676:errorcluster, "VISA out"=w677:refnum<visa-resource-name>)  [unwired: 5 in]
                        }
                        frame True {
                        }
                      }
                      n181 = call "Motors Move Absolute.vi"("Axis Multiplier"=w652, "Axis"=w653, "error in"=w655, "VISA in"=w656, "Position (mm or degree)"=0.0) -> ("error out"=w660:errorcluster, "VISA out"=w661:refnum<visa-resource-name>)  [unwired: 5 in]
                    }
                    frame 2 {
                      w685 = u32 1 ("Axis Multiplier")
                      w687 = 3 ("Axis")
                      n182 = property on="Property Node" class="DigNum (strict)"(reference=w684) -> ("Value"=w686:u32)  [unwired: 1 in, 2 out]
                      n183 = call "Motors Status.vi"("error in"=w697, "VISA in"=w698, "Axis"=w687, "Axis Multiplier"=w686) -> ("error out"=w695:errorcluster, "VISA out"=w696:refnum<visa-resource-name>, "OS"=w705:i32, "Actual Position (mm or deg)"=w701:dbl)  [unwired: 3 in]
                      n184 = property on="Property Node" class="DigNum (strict)"(reference=w683, "Value"=w701) -> ()  [unwired: 1 in, 2 out]
                      n185 = call "Motors Position Redefine.vi"("Axis Multiplier"=w685, "Axis"=w687, "error in"=w695, "VISA in"=w696, "Position (mm or deg)"=w700) -> ("error out"=w693:errorcluster, "VISA out"=w694:refnum<visa-resource-name>)  [unwired: 5 in]
                      n186 = call "Motors Decipher Status.vi"("OS"=w705) -> ("Status"=w703:string)
                      n187 = property on="Property Node" class="Str"(reference=w682, "Value"=w703) -> ()  [unwired: 1 in, 2 out]
                      n188 = Equal?(x=w703, y="Idle") -> (x = y?=w702:bool)
                      n189 = property on="Steps to deactivate hard limit after finding datums" class="DigNum (strict)"() -> ("Value"=w688:dbl)  [unwired: 2 in, 2 out]
                      n190 = case shown="False" w702 {
                        tunnel: w694 -> [w712 w713]
                        tunnel: w693 -> [w711 w714]
                        tunnel: [w710 w713] -> w692
                        tunnel: [w709 w714] -> w691
                        tunnel: w688 -> [w708 _]
                        tunnel: w687 -> [w707 _]
                        tunnel: w685 -> [w706 _]
                        frame False {
                          n191 = call "Motors Move Relative.vi"("Axis Multiplier"=w706, "Axis"=w707, "error in"=w711, "VISA in"=w712, "Distance (mm)"=w708) -> ("error out"=w709:errorcluster, "VISA out"=w710:refnum<visa-resource-name>)  [unwired: 5 in]
                        }
                        frame True {
                        }
                      }
                      n192 = call "Motors Move Absolute.vi"("Axis Multiplier"=w686, "Axis"=w687, "error in"=w691, "VISA in"=w692, "Position (mm or degree)"=0.0) -> ("error out"=w689:errorcluster, "VISA out"=w690:refnum<visa-resource-name>)  [unwired: 5 in]
                    }
                    frame 3 {
                      w718 = u32 1 ("Axis Multiplier")
                      w720 = 4 ("Axis")
                      n193 = property on="Property Node" class="DigNum (strict)"(reference=w717) -> ("Value"=w719:u32)  [unwired: 1 in, 2 out]
                      n194 = call "Motors Status.vi"("error in"=w733, "VISA in"=w734, "Axis"=w720, "Axis Multiplier"=w719) -> ("error out"=w730:errorcluster, "VISA out"=w731:refnum<visa-resource-name>, "OS"=w738:i32, "Actual Position (mm or deg)"=w732:dbl)  [unwired: 3 in]
                      n195 = property on="Property Node" class="DigNum (strict)"(reference=w716, "Value"=w732) -> ()  [unwired: 1 in, 2 out]
                      n196 = call "Motors Position Redefine.vi"("Axis Multiplier"=w718, "Axis"=w720, "error in"=w730, "VISA in"=w731, "Position (mm or deg)"=w729) -> ("error out"=w724:errorcluster, "VISA out"=w725:refnum<visa-resource-name>)  [unwired: 5 in]
                      n197 = call "Motors Decipher Status.vi"("OS"=w738) -> ("Status"=w736:string)
                      n198 = property on="Property Node" class="Str"(reference=w715, "Value"=w736) -> ()  [unwired: 1 in, 2 out]
                      n199 = Equal?(x=w736, y="Idle") -> (x = y?=w735:bool)
                      n200 = case shown="False" w735 {
                        tunnel: w725 -> [w745 w747]
                        tunnel: w724 -> [w744 w746]
                        tunnel: [w743 w747] -> w723
                        tunnel: [w742 w746] -> w722
                        tunnel: "Steps to deactivate hard limit after finding datums" -> [w741 _]
                        tunnel: w720 -> [w740 _]
                        tunnel: w718 -> [w739 _]
                        frame False {
                          n201 = call "Motors Move Relative.vi"("Axis Multiplier"=w739, "Axis"=w740, "error in"=w744, "VISA in"=w745, "Distance (mm)"=w741) -> ("error out"=w742:errorcluster, "VISA out"=w743:refnum<visa-resource-name>)  [unwired: 5 in]
                        }
                        frame True {
                        }
                      }
                      n202 = call "Motors Move Absolute.vi"("Axis Multiplier"=w719, "Axis"=w720, "error in"=w722, "VISA in"=w723, "Position (mm or degree)"=0.0) -> ("error out"=w726:errorcluster, "VISA out"=w727:refnum<visa-resource-name>)  [unwired: 5 in]
                    }
                  }
                }
              }
              frame #2 {
                n203 = call <vilib>:"Unset Busy.vi"() -> ()  [unwired: 11 in, 1 out]
                n204 = property on="Property Node" class="Str"(reference=w749, "Value"="Running" ("Status")) -> (reference out=w748:refnum<vi>)  [unwired: 1 in, 1 out]
              }
            }
          }
        }
        n205 = Unbundle(w245) -> ("X Go?"=w244:refnum<vi>, "X Multiplier"=w243:refnum<vi>, "X Go To"=w242:refnum<vi>, "Y Go?"=w241:refnum<vi>, "Y Multiplier"=w240:refnum<vi>, "Y Go To"=w239:refnum<vi>, "Z Go?"=w238:refnum<vi>, "Z Multiplier"=w237:refnum<vi>, "Z Go To"=w236:refnum<vi>, "Theta Go?"=w235:refnum<vi>, "Theta Multiplier"=w234:refnum<vi>, "Theta Go To"=w233:refnum<vi>)
        n206 = property on="Property Node" class="Bool (strict)"(reference=w244) -> (reference out=w348:refnum<vi>, "Value"=w361:bool)  [unwired: 1 in, 1 out]
        n207 = case shown="True" w361 {
          tunnel: w371 -> [w1642 w1650]
          tunnel: w373 -> [w1641 w1653]
          tunnel: [w1642 w1651] -> w419
          tunnel: [w1641 w1652] -> w418
          tunnel: w348 -> [_ w1648]
          tunnel: w243 -> [_ w1644]
          tunnel: w242 -> [_ w1643]
          frame False {
          }
          frame True {
            n208 = property on="Property Node" class="DigNum (strict)"(reference=w1644) -> ("Value"=w1646:u32)  [unwired: 1 in, 2 out]
            n209 = property on="Property Node" class="DigNum (strict)"(reference=w1643) -> ("Value"=w1645:dbl)  [unwired: 1 in, 2 out]
            n210 = property on="Property Node" class="Bool (strict)"(reference=w1648, "Value"=FALSE) -> ()  [unwired: 1 in, 2 out]
            n211 = call "Motors Move Absolute.vi"("Axis Multiplier"=w1646, "Axis"=u32 1, "error in"=w1653, "VISA in"=w1650, "Position (mm or degree)"=w1645) -> ("error out"=w1652:errorcluster, "VISA out"=w1651:refnum<visa-resource-name>)  [unwired: 5 in]
          }
        }
        n212 = property on="Property Node" class="Bool (strict)"(reference=w241) -> (reference out=w353:refnum<vi>, "Value"=w354:bool)  [unwired: 1 in, 1 out]
        n213 = case shown="True" w354 {
          tunnel: w419 -> [w1629 w1637]
          tunnel: w418 -> [w1628 w1640]
          tunnel: [w1629 w1638] -> w417
          tunnel: [w1628 w1639] -> w416
          tunnel: w353 -> [_ w1632]
          tunnel: w240 -> [_ w1631]
          tunnel: w239 -> [_ w1630]
          frame False {
          }
          frame True {
            n214 = property on="Property Node" class="DigNum (strict)"(reference=w1631) -> ("Value"=w1635:u32)  [unwired: 1 in, 2 out]
            n215 = property on="Property Node" class="DigNum (strict)"(reference=w1630) -> ("Value"=w1634:dbl)  [unwired: 1 in, 2 out]
            n216 = property on="Property Node" class="Bool (strict)"(reference=w1632, "Value"=FALSE) -> ()  [unwired: 1 in, 2 out]
            n217 = call "Motors Move Absolute.vi"("Axis Multiplier"=w1635, "Axis"=u32 2, "error in"=w1640, "VISA in"=w1637, "Position (mm or degree)"=w1634) -> ("error out"=w1639:errorcluster, "VISA out"=w1638:refnum<visa-resource-name>)  [unwired: 5 in]
          }
        }
        n218 = property on="Property Node" class="Bool (strict)"(reference=w238) -> (reference out=w351:refnum<vi>, "Value"=w352:bool)  [unwired: 1 in, 1 out]
        n219 = case shown="True" w352 {
          tunnel: w417 -> [w1616 w1622]
          tunnel: w416 -> [w1615 w1627]
          tunnel: [w1616 w1625] -> w415
          tunnel: [w1615 w1626] -> w414
          tunnel: w351 -> [_ w1619]
          tunnel: w237 -> [_ w1618]
          tunnel: w236 -> [_ w1617]
          frame False {
          }
          frame True {
            n220 = property on="Property Node" class="DigNum (strict)"(reference=w1618) -> ("Value"=w1623:u32)  [unwired: 1 in, 2 out]
            n221 = property on="Property Node" class="DigNum (strict)"(reference=w1617) -> ("Value"=w1621:dbl)  [unwired: 1 in, 2 out]
            n222 = property on="Property Node" class="Bool (strict)"(reference=w1619, "Value"=FALSE) -> ()  [unwired: 1 in, 2 out]
            n223 = call "Motors Move Absolute.vi"("Axis Multiplier"=w1623, "Axis"=u32 3, "error in"=w1627, "VISA in"=w1622, "Position (mm or degree)"=w1621) -> ("error out"=w1626:errorcluster, "VISA out"=w1625:refnum<visa-resource-name>)  [unwired: 5 in]
          }
        }
        n224 = property on="Property Node" class="Bool (strict)"(reference=w235) -> (reference out=w349:refnum<vi>, "Value"=w350:bool)  [unwired: 1 in, 1 out]
        n225 = case shown="True" w350 {
          tunnel: w415 -> [w1602 w1611]
          tunnel: w414 -> [w1603 w1614]
          tunnel: [w1603 w1613] -> w412
          tunnel: [w1602 w1612] -> w413
          tunnel: w349 -> [_ w1606]
          tunnel: w234 -> [_ w1605]
          tunnel: w233 -> [_ w1604]
          frame False {
          }
          frame True {
            n226 = property on="Property Node" class="DigNum (strict)"(reference=w1605) -> ("Value"=w1609:u32)  [unwired: 1 in, 2 out]
            n227 = property on="Property Node" class="DigNum (strict)"(reference=w1604) -> ("Value"=w1608:dbl)  [unwired: 1 in, 2 out]
            n228 = property on="Property Node" class="Bool (strict)"(reference=w1606, "Value"=FALSE) -> ()  [unwired: 1 in, 2 out]
            n229 = call "Motors Move Absolute.vi"("Axis Multiplier"=w1609, "Axis"=u32 4, "error in"=w1614, "VISA in"=w1611, "Position (mm or degree)"=w1608) -> ("error out"=w1613:errorcluster, "VISA out"=w1612:refnum<visa-resource-name>)  [unwired: 5 in]
          }
        }
        n230 = Unbundle(w232) -> ("Jog-Mode"=w229:refnum<vi>, "x+?"=w230:refnum<vi>, "x-?"=w231:refnum<vi>, "X Moving"=w220:refnum<vi>, "X Multiplier"=w225:refnum<vi>, "Delta X (mm)"=w219:refnum<vi>, "X Speed (mm/s)"=w226:refnum<vi>, "x+"=w222:refnum<vi>, "x-"=w221:refnum<vi>, "X-Axis (mm)"=w224:refnum<vi>, "Status X"=w223:refnum<vi>)
        n231 = property on="Property Node" class="Bool (strict)"(reference=w229) -> ("Value"=w227:bool)  [unwired: 1 in, 2 out]
        n232 = property on="Property Node" class="Bool (strict)"(reference=w230) -> (reference out=w346:refnum<vi>, "Value"=w384:bool)  [unwired: 1 in, 1 out]
        n233 = property on="Property Node" class="Bool (strict)"(reference=w231) -> (reference out=w347:refnum<vi>, "Value"=w383:bool)  [unwired: 1 in, 1 out]
        n234 = Or(x=w384, y=w383) -> (x .or. y?=w411:bool)
        n235 = case shown="True" w411 {
          tunnel: w413 -> [w1495 w1512]
          tunnel: w412 -> [w1494 w1511]
          tunnel: w227 -> [_ w1513]
          tunnel: [w1495 w1509] -> w410
          tunnel: [w1494 w1508] -> w409
          tunnel: w383 -> [_ w1510]
          tunnel: w347 -> [_ w1505]
          tunnel: w346 -> [_ w1504]
          tunnel: w226 -> [_ w1503]
          tunnel: w225 -> [_ w1502]
          tunnel: w224 -> [_ w1501]
          tunnel: w223 -> [_ w1500]
          tunnel: w222 -> [_ w1499]
          tunnel: w221 -> [_ w1498]
          tunnel: w220 -> [_ w1497]
          tunnel: w219 -> [_ w1496]
          frame False {
          }
          frame True {
            n236 = flat-sequence {
              tunnel: w1513 -> [w1527]
              tunnel: w1512 -> [w1526]
              tunnel: w1511 -> [w1525]
              tunnel: w1510 -> [w1524]
              tunnel: [w1523] -> w1507
              tunnel: [w1522] -> w1506
              tunnel: w1503 -> [w1521]
              tunnel: w1502 -> [w1520]
              tunnel: w1501 -> [w1519]
              tunnel: w1500 -> [w1518]
              tunnel: w1499 -> [w1517]
              tunnel: w1498 -> [w1516]
              tunnel: w1497 -> [w1515]
              tunnel: w1496 -> [w1514]
              tunnel: [w1600] -> w1508
              tunnel: [w1601] -> w1509
              tunnel: w1507 -> [w1601]
              tunnel: w1506 -> [w1600]
              tunnel: w1505 -> [w1597]
              tunnel: w1504 -> [w1596]
              frame #0 {
                n237 = case shown="False" w1527 {
                  tunnel: w1526 -> [w1537 w1567]
                  tunnel: w1525 -> [w1533 w1570]
                  tunnel: w1524 -> [w1536 w1575]
                  tunnel: [w1535 w1572] -> w1523
                  tunnel: [w1534 w1571] -> w1522
                  tunnel: w1521 -> [_ w1562]
                  tunnel: w1520 -> [w1528 w1561]
                  tunnel: w1519 -> [_ w1560]
                  tunnel: w1518 -> [_ w1559]
                  tunnel: w1517 -> [_ w1558]
                  tunnel: w1516 -> [_ w1557]
                  tunnel: w1515 -> [w1530 _]
                  tunnel: w1514 -> [w1529 _]
                  frame False {
                    n238 = property on="Property Node" class="Bool (strict)"(reference=w1530) -> (reference out=w1531:refnum<vi>, "Value"=w1532:bool)  [unwired: 1 in, 1 out]
                    n239 = case shown="False" w1532 {
                      tunnel: w1537 -> [w1545 w1556]
                      tunnel: w1533 -> [w1550 w1555]
                      tunnel: w1536 -> [w1549 _]
                      tunnel: [w1547 w1556] -> w1535
                      tunnel: [w1548 w1555] -> w1534
                      tunnel: w1531 -> [w1541 _]
                      tunnel: w1529 -> [w1539 _]
                      tunnel: w1528 -> [w1538 _]
                      frame False {
                        n240 = property on="Property Node" class="Bool (strict)"(reference=w1541, "Value"=TRUE ("X Moving")) -> ()  [unwired: 1 in, 2 out]
                        n241 = property on="Property Node" class="DigNum (strict)"(reference=w1538) -> ("Value"=w1543:u32)  [unwired: 1 in, 2 out]
                        n242 = property on="Property Node" class="DigNum (strict)"(reference=w1539) -> ("Value"=w1540:dbl)  [unwired: 1 in, 2 out]
                        n243 = case shown="True" w1549 {
                          tunnel: w1540 -> [w1551 w1553]
                          tunnel: [w1551 w1552] -> w1546
                          frame False {
                          }
                          frame True {
                            n244 = Multiply(x=w1553, y=-1.0) -> (x*y=w1552:dbl)
                          }
                        }
                        n245 = call "Motors Move Relative.vi"("Axis Multiplier"=w1543, "Axis"=1, "error in"=w1550, "VISA in"=w1545, "Distance (mm)"=w1546) -> ("error out"=w1548:errorcluster, "VISA out"=w1547:refnum<visa-resource-name>)  [unwired: 5 in]
                      }
                      frame True {
                      }
                    }
                  }
                  frame True {
                    w1564 = 1 ("Axis")
                    n246 = property on="Property Node" class="DigNum (strict)"(reference=w1561) -> ("Value"=w1565:u32)  [unwired: 1 in, 2 out]
                    n247 = property on="Property Node" class="DigNum (strict)"(reference=w1562) -> ("Value"=w1563:dbl)  [unwired: 1 in, 2 out]
                    n248 = case shown="True" w1575 {
                      tunnel: w1563 -> [w1592 w1594]
                      tunnel: [w1592 w1593] -> w1568
                      frame False {
                      }
                      frame True {
                        n249 = Multiply(x=w1594, y=-1.0) -> (x*y=w1593:dbl)
                      }
                    }
                    n250 = call "Motors Move Constant Velocity.vi"("Axis Multiplier"=w1565, "Axis"=w1564, "error in"=w1570, "VISA in"=w1567, "Speed (mm/s)"=w1568) -> ("error out"=w1569:errorcluster, "VISA out"=w1566:refnum<visa-resource-name>)  [unwired: 5 in]
                    n251 = while {
                      tunnel: w1566 -> [w1581]
                      tunnel: [w1583] -> w1574
                      tunnel: w1569 -> [w1584]
                      tunnel: [w1582] -> w1573
                      tunnel: w1565 -> [w1580]
                      tunnel: w1560 -> [w1579]
                      tunnel: w1559 -> [w1578]
                      tunnel: w1558 -> [w1577]
                      tunnel: w1557 -> [w1576]
                      stop <- w1589 continue-if-true
                      n252 = property on="Property Node" class="Bool (strict)"(reference=w1577) -> ("Value"=w1590:bool)  [unwired: 1 in, 2 out]
                      n253 = property on="Property Node" class="Bool (strict)"(reference=w1576) -> ("Value"=w1591:bool)  [unwired: 1 in, 2 out]
                      n254 = Or(x=w1590, y=w1591) -> (x .or. y?=w1589:bool)
                      n255 = call "Motors Status.vi"("error in"=w1584, "VISA in"=w1581, "Axis"=1, "Axis Multiplier"=w1580) -> ("error out"=w1582:errorcluster, "VISA out"=w1583:refnum<visa-resource-name>, "OS"=w1587:i32, "Actual Position (mm or deg)"=w1585:dbl)  [unwired: 3 in]
                      n256 = property on="Property Node" class="DigNum (strict)"(reference=w1579, "Value"=w1585) -> ()  [unwired: 1 in, 2 out]
                      n257 = call "Motors Decipher Status.vi"("OS"=w1587) -> ("Status"=w1586:string)
                      n258 = property on="Property Node" class="Str"(reference=w1578, "Value"=w1586) -> ()  [unwired: 1 in, 2 out]
                    }
                    n259 = call "Motors Stop.vi"("error in"=w1573, "Axis"=w1564, "VISA in"=w1574) -> ("error out"=w1571:errorcluster, "VISA out"=w1572:refnum<visa-resource-name>)
                  }
                }
              }
              frame #1 {
                n260 = property on="Property Node" class="Bool (strict)"(reference=w1596, "Value"=FALSE) -> ()  [unwired: 1 in, 2 out]
                n261 = property on="Property Node" class="Bool (strict)"(reference=w1597, "Value"=FALSE) -> ()  [unwired: 1 in, 2 out]
              }
            }
          }
        }
        n262 = Unbundle(w218) -> ("Jog-Mode"=w217:refnum<vi>, "y+?"=w205:refnum<vi>, "y-?"=w204:refnum<vi>, "Y Moving"=w207:refnum<vi>, "Delta Y (mm)"=w206:refnum<vi>, "Y Multiplier"=w214:refnum<vi>, "y+"=w213:refnum<vi>, "y-"=w212:refnum<vi>, "Y-Axis (mm)"=w210:refnum<vi>, "Status Y"=w211:refnum<vi>, "Y Speed (mm/s)"=w215:refnum<vi>)
        n263 = property on="Property Node" class="Bool (strict)"(reference=w217) -> ("Value"=w216:bool)  [unwired: 1 in, 2 out]
        n264 = property on="Property Node" class="Bool (strict)"(reference=w205) -> (reference out=w209:refnum<vi>, "Value"=w382:bool)  [unwired: 1 in, 1 out]
        n265 = property on="Property Node" class="Bool (strict)"(reference=w204) -> (reference out=w208:refnum<vi>, "Value"=w381:bool)  [unwired: 1 in, 1 out]
        n266 = Or(x=w382, y=w381) -> (x .or. y?=w408:bool)
        n267 = case shown="True" w408 {
          tunnel: w410 -> [w1387 w1404]
          tunnel: w409 -> [w1386 w1403]
          tunnel: w216 -> [_ w1405]
          tunnel: [w1387 w1402] -> w407
          tunnel: [w1386 w1401] -> w406
          tunnel: w381 -> [_ w1400]
          tunnel: w215 -> [_ w1397]
          tunnel: w214 -> [_ w1396]
          tunnel: w213 -> [_ w1395]
          tunnel: w212 -> [_ w1394]
          tunnel: w211 -> [_ w1393]
          tunnel: w210 -> [_ w1392]
          tunnel: w209 -> [_ w1391]
          tunnel: w208 -> [_ w1390]
          tunnel: w207 -> [_ w1389]
          tunnel: w206 -> [_ w1388]
          frame False {
          }
          frame True {
            n268 = flat-sequence {
              tunnel: w1405 -> [w1419]
              tunnel: w1404 -> [w1418]
              tunnel: w1403 -> [w1417]
              tunnel: w1400 -> [w1414]
              tunnel: [w1416] -> w1399
              tunnel: [w1415] -> w1398
              tunnel: w1397 -> [w1413]
              tunnel: w1396 -> [w1412]
              tunnel: w1395 -> [w1411]
              tunnel: w1394 -> [w1410]
              tunnel: w1393 -> [w1409]
              tunnel: w1392 -> [w1408]
              tunnel: w1389 -> [w1407]
              tunnel: w1388 -> [w1406]
              tunnel: [w1492] -> w1401
              tunnel: [w1493] -> w1402
              tunnel: w1399 -> [w1493]
              tunnel: w1398 -> [w1492]
              tunnel: w1391 -> [w1489]
              tunnel: w1390 -> [w1488]
              frame #0 {
                n269 = case shown="False" w1419 {
                  tunnel: w1418 -> [w1429 w1459]
                  tunnel: w1417 -> [w1428 w1462]
                  tunnel: [w1427 w1465] -> w1416
                  tunnel: [w1426 w1464] -> w1415
                  tunnel: w1414 -> [w1425 w1463]
                  tunnel: w1413 -> [_ w1454]
                  tunnel: w1412 -> [w1423 w1453]
                  tunnel: w1411 -> [_ w1452]
                  tunnel: w1410 -> [_ w1451]
                  tunnel: w1409 -> [_ w1450]
                  tunnel: w1408 -> [_ w1449]
                  tunnel: w1407 -> [w1422 _]
                  tunnel: w1406 -> [w1420 _]
                  frame False {
                    n270 = property on="Property Node" class="Bool (strict)"(reference=w1422) -> (reference out=w1421:refnum<vi>, "Value"=w1424:bool)  [unwired: 1 in, 1 out]
                    n271 = case shown="False" w1424 {
                      tunnel: w1429 -> [w1438 w1448]
                      tunnel: w1428 -> [w1442 w1447]
                      tunnel: [w1439 w1448] -> w1427
                      tunnel: [w1441 w1447] -> w1426
                      tunnel: w1425 -> [w1440 _]
                      tunnel: w1423 -> [w1433 _]
                      tunnel: w1421 -> [w1432 _]
                      tunnel: w1420 -> [w1431 _]
                      frame False {
                        n272 = property on="Property Node" class="Bool (strict)"(reference=w1432, "Value"=TRUE ("Y Moving")) -> ()  [unwired: 1 in, 2 out]
                        n273 = property on="Property Node" class="DigNum (strict)"(reference=w1431) -> ("Value"=w1430:dbl)  [unwired: 1 in, 2 out]
                        n274 = property on="Property Node" class="DigNum (strict)"(reference=w1433) -> ("Value"=w1435:u32)  [unwired: 1 in, 2 out]
                        n275 = case shown="True" w1440 {
                          tunnel: w1430 -> [w1443 w1445]
                          tunnel: [w1443 w1444] -> w1437
                          frame False {
                          }
                          frame True {
                            n276 = Multiply(x=w1445, y=-1.0) -> (x*y=w1444:dbl)
                          }
                        }
                        n277 = call "Motors Move Relative.vi"("Axis Multiplier"=w1435, "Axis"=2, "error in"=w1442, "VISA in"=w1438, "Distance (mm)"=w1437) -> ("error out"=w1441:errorcluster, "VISA out"=w1439:refnum<visa-resource-name>)  [unwired: 5 in]
                      }
                      frame True {
                      }
                    }
                  }
                  frame True {
                    w1456 = 2 ("Axis")
                    n278 = property on="Property Node" class="DigNum (strict)"(reference=w1453) -> ("Value"=w1457:u32)  [unwired: 1 in, 2 out]
                    n279 = property on="Property Node" class="DigNum (strict)"(reference=w1454) -> ("Value"=w1455:dbl)  [unwired: 1 in, 2 out]
                    n280 = case shown="True" w1463 {
                      tunnel: w1455 -> [w1484 w1486]
                      tunnel: [w1484 w1485] -> w1460
                      frame False {
                      }
                      frame True {
                        n281 = Multiply(x=w1486, y=-1.0) -> (x*y=w1485:dbl)
                      }
                    }
                    n282 = call "Motors Move Constant Velocity.vi"("Axis Multiplier"=w1457, "Axis"=w1456, "error in"=w1462, "VISA in"=w1459, "Speed (mm/s)"=w1460) -> ("error out"=w1461:errorcluster, "VISA out"=w1458:refnum<visa-resource-name>)  [unwired: 5 in]
                    n283 = while {
                      tunnel: w1458 -> [w1474]
                      tunnel: [w1473] -> w1467
                      tunnel: w1461 -> [w1476]
                      tunnel: [w1475] -> w1466
                      tunnel: w1457 -> [w1472]
                      tunnel: w1452 -> [w1471]
                      tunnel: w1451 -> [w1470]
                      tunnel: w1450 -> [w1469]
                      tunnel: w1449 -> [w1468]
                      stop <- w1483 continue-if-true
                      n284 = property on="Property Node" class="Bool (strict)"(reference=w1471) -> ("Value"=w1482:bool)  [unwired: 1 in, 2 out]
                      n285 = property on="Property Node" class="Bool (strict)"(reference=w1470) -> ("Value"=w1481:bool)  [unwired: 1 in, 2 out]
                      n286 = Or(x=w1482, y=w1481) -> (x .or. y?=w1483:bool)
                      n287 = call "Motors Status.vi"("error in"=w1476, "VISA in"=w1474, "Axis"=2, "Axis Multiplier"=w1472) -> ("error out"=w1475:errorcluster, "VISA out"=w1473:refnum<visa-resource-name>, "OS"=w1478:i32, "Actual Position (mm or deg)"=w1479:dbl)  [unwired: 3 in]
                      n288 = property on="Property Node" class="DigNum (strict)"(reference=w1468, "Value"=w1479) -> ()  [unwired: 1 in, 2 out]
                      n289 = call "Motors Decipher Status.vi"("OS"=w1478) -> ("Status"=w1477:string)
                      n290 = property on="Property Node" class="Str"(reference=w1469, "Value"=w1477) -> ()  [unwired: 1 in, 2 out]
                    }
                    n291 = call "Motors Stop.vi"("error in"=w1466, "Axis"=w1456, "VISA in"=w1467) -> ("error out"=w1464:errorcluster, "VISA out"=w1465:refnum<visa-resource-name>)
                  }
                }
              }
              frame #1 {
                n292 = property on="Property Node" class="Bool (strict)"(reference=w1489, "Value"=FALSE) -> ()  [unwired: 1 in, 2 out]
                n293 = property on="Property Node" class="Bool (strict)"(reference=w1488, "Value"=FALSE) -> ()  [unwired: 1 in, 2 out]
              }
            }
          }
        }
        n294 = Unbundle(w203) -> ("Jog-Mode"=w200:refnum<vi>, "z+?"=w202:refnum<vi>, "z-?"=w201:refnum<vi>, "Z Speed (mm/s)"=w195:refnum<vi>, "Delta Z (mm)"=w197:refnum<vi>, "Z Multiplier"=w196:refnum<vi>, "Z-Axis (mm)"=w192:refnum<vi>, "Status Z"=w191:refnum<vi>, "z+"=w194:refnum<vi>, "z-"=w193:refnum<vi>, "Z Moving"=w198:refnum<vi>)
        n295 = property on="Property Node" class="Bool (strict)"(reference=w202) -> (reference out=w344:refnum<vi>, "Value"=w379:bool)  [unwired: 1 in, 1 out]
        n296 = property on="Property Node" class="Bool (strict)"(reference=w201) -> (reference out=w345:refnum<vi>, "Value"=w380:bool)  [unwired: 1 in, 1 out]
        n297 = property on="Property Node" class="Bool (strict)"(reference=w200) -> ("Value"=w199:bool)  [unwired: 1 in, 2 out]
        n298 = Or(x=w379, y=w380) -> (x .or. y?=w405:bool)
        n299 = case shown="True" w405 {
          tunnel: w407 -> [w1275 w1293]
          tunnel: w406 -> [w1274 w1287]
          tunnel: w199 -> [_ w1294]
          tunnel: [w1275 w1292] -> w402
          tunnel: [w1274 w1291] -> w403
          tunnel: w380 -> [_ w1290]
          tunnel: w345 -> [_ w1286]
          tunnel: w345 -> [_ w1285]
          tunnel: w344 -> [_ w1284]
          tunnel: w198 -> [_ w1283]
          tunnel: w197 -> [_ w1282]
          tunnel: w196 -> [_ w1281]
          tunnel: w195 -> [_ w1280]
          tunnel: w194 -> [_ w1279]
          tunnel: w193 -> [_ w1278]
          tunnel: w192 -> [_ w1277]
          tunnel: w191 -> [_ w1276]
          frame False {
          }
          frame True {
            n300 = flat-sequence {
              tunnel: w1294 -> [w1309]
              tunnel: w1293 -> [w1308]
              tunnel: w1290 -> [w1305]
              tunnel: [w1307] -> w1289
              tunnel: [w1306] -> w1288
              tunnel: w1287 -> [w1304]
              tunnel: w1286 -> [w1303]
              tunnel: w1283 -> [w1302]
              tunnel: w1282 -> [w1301]
              tunnel: w1281 -> [w1300]
              tunnel: w1280 -> [w1299]
              tunnel: w1279 -> [w1298]
              tunnel: w1278 -> [w1297]
              tunnel: w1277 -> [w1296]
              tunnel: w1276 -> [w1295]
              tunnel: [w1384] -> w1291
              tunnel: [w1385] -> w1292
              tunnel: w1289 -> [w1385]
              tunnel: w1288 -> [w1384]
              tunnel: w1285 -> [w1381]
              tunnel: w1284 -> [w1380]
              frame #0 {
                n301 = case shown="True" w1309 {
                  tunnel: w1308 -> [w1319 w1351]
                  tunnel: w1304 -> [w1318 w1354]
                  tunnel: [w1317 w1357] -> w1307
                  tunnel: [w1316 w1356] -> w1306
                  tunnel: w1305 -> [w1315 w1346]
                  tunnel: w1304 -> [_ w1348]
                  tunnel: w1303 -> [_ w1345]
                  tunnel: w1302 -> [w1312 _]
                  tunnel: w1301 -> [w1311 _]
                  tunnel: w1300 -> [w1310 w1344]
                  tunnel: w1299 -> [_ w1343]
                  tunnel: w1298 -> [_ w1342]
                  tunnel: w1297 -> [_ w1341]
                  tunnel: w1296 -> [_ w1340]
                  tunnel: w1295 -> [_ w1339]
                  frame False {
                    n302 = property on="Property Node" class="Bool (strict)"(reference=w1312) -> (reference out=w1313:refnum<vi>, "Value"=w1314:bool)  [unwired: 1 in, 1 out]
                    n303 = case shown="False" w1314 {
                      tunnel: w1319 -> [w1325 w1338]
                      tunnel: w1318 -> [w1332 w1337]
                      tunnel: [w1326 w1338] -> w1317
                      tunnel: [w1331 w1337] -> w1316
                      tunnel: w1315 -> [w1330 _]
                      tunnel: w1313 -> [w1322 _]
                      tunnel: w1311 -> [w1321 _]
                      tunnel: w1310 -> [w1320 _]
                      frame False {
                        n304 = property on="Property Node" class="Bool (strict)"(reference=w1322, "Value"=TRUE ("Z Moving")) -> ()  [unwired: 1 in, 2 out]
                        n305 = property on="Property Node" class="DigNum (strict)"(reference=w1321) -> ("Value"=w1323:dbl)  [unwired: 1 in, 2 out]
                        n306 = property on="Property Node" class="DigNum (strict)"(reference=w1320) -> ("Value"=w1328:u32)  [unwired: 1 in, 2 out]
                        n307 = case shown="True" w1330 {
                          tunnel: w1323 -> [w1333 w1335]
                          tunnel: [w1333 w1334] -> w1327
                          frame False {
                          }
                          frame True {
                            n308 = Multiply(x=w1335, y=-1.0) -> (x*y=w1334:dbl)
                          }
                        }
                        n309 = call "Motors Move Relative.vi"("Axis Multiplier"=w1328, "Axis"=3, "error in"=w1332, "VISA in"=w1325, "Distance (mm)"=w1327) -> ("error out"=w1331:errorcluster, "VISA out"=w1326:refnum<visa-resource-name>)  [unwired: 5 in]
                      }
                      frame True {
                      }
                    }
                  }
                  frame True {
                    w1353 = 3 ("Axis")
                    n310 = property on="Property Node" class="DigNum (strict)"(reference=w1343, error in=w1348) -> ("Value"=w1347:dbl)  [unwired: 2 out]
                    n311 = property on="Property Node" class="DigNum (strict)"(reference=w1344) -> ("Value"=w1349:u32)  [unwired: 1 in, 2 out]
                    n312 = case shown="True" w1346 {
                      tunnel: w1347 -> [w1376 w1378]
                      tunnel: [w1376 w1377] -> w1352
                      frame False {
                      }
                      frame True {
                        n313 = Multiply(x=w1378, y=-1.0) -> (x*y=w1377:dbl)
                      }
                    }
                    n314 = call "Motors Move Constant Velocity.vi"("Axis Multiplier"=w1349, "Axis"=w1353, "error in"=w1354, "VISA in"=w1351, "Speed (mm/s)"=w1352) -> ("error out"=w1355:errorcluster, "VISA out"=w1350:refnum<visa-resource-name>)  [unwired: 5 in]
                    n315 = while {
                      tunnel: w1350 -> [w1366]
                      tunnel: [w1365] -> w1359
                      tunnel: w1355 -> [w1368]
                      tunnel: [w1367] -> w1358
                      tunnel: w1349 -> [w1364]
                      tunnel: w1345 -> [_]
                      tunnel: w1342 -> [w1363]
                      tunnel: w1341 -> [w1362]
                      tunnel: w1340 -> [w1361]
                      tunnel: w1339 -> [w1360]
                      stop <- w1375 continue-if-true
                      n316 = property on="Property Node" class="Bool (strict)"(reference=w1363) -> ("Value"=w1374:bool)  [unwired: 1 in, 2 out]
                      n317 = property on="Property Node" class="Bool (strict)"(reference=w1362) -> ("Value"=w1373:bool)  [unwired: 1 in, 2 out]
                      n318 = Or(x=w1374, y=w1373) -> (x .or. y?=w1375:bool)
                      n319 = call "Motors Status.vi"("error in"=w1368, "VISA in"=w1366, "Axis"=3, "Axis Multiplier"=w1364) -> ("error out"=w1367:errorcluster, "VISA out"=w1365:refnum<visa-resource-name>, "OS"=w1370:i32, "Actual Position (mm or deg)"=w1371:dbl)  [unwired: 3 in]
                      n320 = property on="Property Node" class="DigNum (strict)"(reference=w1361, "Value"=w1371) -> ()  [unwired: 1 in, 2 out]
                      n321 = call "Motors Decipher Status.vi"("OS"=w1370) -> ("Status"=w1369:string)
                      n322 = property on="Property Node" class="Str"(reference=w1360, "Value"=w1369) -> ()  [unwired: 1 in, 2 out]
                    }
                    n323 = call "Motors Stop.vi"("error in"=w1358, "Axis"=w1353, "VISA in"=w1359) -> ("error out"=w1356:errorcluster, "VISA out"=w1357:refnum<visa-resource-name>)
                  }
                }
              }
              frame #1 {
                n324 = property on="Property Node" class="Bool (strict)"(reference=w1380, "Value"=FALSE) -> ()  [unwired: 1 in, 2 out]
                n325 = property on="Property Node" class="Bool (strict)"(reference=w1381, "Value"=FALSE) -> ()  [unwired: 1 in, 2 out]
              }
            }
          }
        }
        n326 = Unbundle(w190) -> ("Jog-Mode"=w189:refnum<vi>, "theta+?"=w188:refnum<vi>, "theta-?"=w187:refnum<vi>, "Theta Speed (deg/s)"=w183:refnum<vi>, "Delta Theta (deg)"=w177:refnum<vi>, "Theta Multiplier"=w184:refnum<vi>, "Theta (deg)"=w180:refnum<vi>, "Status Theta"=w179:refnum<vi>, "theta+"=w182:refnum<vi>, "theta-"=w181:refnum<vi>, "Theta Moving"=w178:refnum<vi>)
        n327 = property on="Property Node" class="Bool (strict)"(reference=w188) -> (reference out=w185:refnum<vi>, "Value"=w378:bool)  [unwired: 1 in, 1 out]
        n328 = property on="Property Node" class="Bool (strict)"(reference=w187) -> (reference out=w186:refnum<vi>, "Value"=w377:bool)  [unwired: 1 in, 1 out]
        n329 = property on="Property Node" class="Bool (strict)"(reference=w189) -> ("Value"=w228:bool)  [unwired: 1 in, 2 out]
        n330 = Or(x=w378, y=w377) -> (x .or. y?=w404:bool)
        n331 = case shown="True" w404 {
          tunnel: w402 -> [w1167 w1184]
          tunnel: w403 -> [w1166 w1183]
          tunnel: w228 -> [_ w1185]
          tunnel: [w1167 w1182] -> w401
          tunnel: [w1166 w1181] -> w394
          tunnel: w377 -> [_ w1180]
          tunnel: w186 -> [_ w1177]
          tunnel: w185 -> [_ w1176]
          tunnel: w184 -> [_ w1175]
          tunnel: w183 -> [_ w1174]
          tunnel: w182 -> [_ w1173]
          tunnel: w181 -> [_ w1172]
          tunnel: w180 -> [_ w1171]
          tunnel: w179 -> [_ w1170]
          tunnel: w178 -> [_ w1169]
          tunnel: w177 -> [_ w1168]
          frame False {
          }
          frame True {
            n332 = flat-sequence {
              tunnel: w1185 -> [w1199]
              tunnel: w1184 -> [w1198]
              tunnel: w1183 -> [w1197]
              tunnel: w1180 -> [w1194]
              tunnel: [w1196] -> w1179
              tunnel: [w1195] -> w1178
              tunnel: w1175 -> [w1193]
              tunnel: w1174 -> [w1192]
              tunnel: w1173 -> [w1191]
              tunnel: w1172 -> [w1190]
              tunnel: w1171 -> [w1189]
              tunnel: w1170 -> [w1188]
              tunnel: w1169 -> [w1187]
              tunnel: w1168 -> [w1186]
              tunnel: [w1272] -> w1181
              tunnel: [w1273] -> w1182
              tunnel: w1179 -> [w1273]
              tunnel: w1178 -> [w1272]
              tunnel: w1177 -> [w1269]
              tunnel: w1176 -> [w1268]
              frame #0 {
                n333 = case shown="False" w1199 {
                  tunnel: w1198 -> [w1209 w1240]
                  tunnel: w1197 -> [w1208 w1241]
                  tunnel: [w1207 w1245] -> w1196
                  tunnel: [w1206 w1244] -> w1195
                  tunnel: w1194 -> [w1205 w1243]
                  tunnel: w1193 -> [w1203 w1235]
                  tunnel: w1192 -> [_ w1233]
                  tunnel: w1191 -> [_ w1232]
                  tunnel: w1190 -> [_ w1231]
                  tunnel: w1189 -> [_ w1230]
                  tunnel: w1188 -> [_ w1229]
                  tunnel: w1187 -> [w1202 _]
                  tunnel: w1186 -> [w1200 _]
                  frame False {
                    n334 = property on="Property Node" class="Bool (strict)"(reference=w1202) -> (reference out=w1201:refnum<vi>, "Value"=w1204:bool)  [unwired: 1 in, 1 out]
                    n335 = case shown="False" w1204 {
                      tunnel: w1209 -> [w1216 w1228]
                      tunnel: w1208 -> [w1222 w1227]
                      tunnel: [w1217 w1228] -> w1207
                      tunnel: [w1221 w1227] -> w1206
                      tunnel: w1205 -> [w1220 _]
                      tunnel: w1203 -> [w1213 _]
                      tunnel: w1201 -> [w1212 _]
                      tunnel: w1200 -> [w1211 _]
                      frame False {
                        n336 = property on="Property Node" class="Bool (strict)"(reference=w1212, "Value"=TRUE ("Theta Moving")) -> ()  [unwired: 1 in, 2 out]
                        n337 = property on="Property Node" class="DigNum (strict)"(reference=w1211) -> ("Value"=w1210:dbl)  [unwired: 1 in, 2 out]
                        n338 = property on="Property Node" class="DigNum (strict)"(reference=w1213) -> ("Value"=w1219:u32)  [unwired: 1 in, 2 out]
                        n339 = case shown="True" w1220 {
                          tunnel: w1210 -> [w1223 w1225]
                          tunnel: [w1223 w1224] -> w1215
                          frame False {
                          }
                          frame True {
                            n340 = Multiply(x=w1225, y=-1.0) -> (x*y=w1224:dbl)
                          }
                        }
                        n341 = call "Motors Move Relative.vi"("Axis Multiplier"=w1219, "Axis"=4, "error in"=w1222, "VISA in"=w1216, "Distance (mm)"=w1215) -> ("error out"=w1221:errorcluster, "VISA out"=w1217:refnum<visa-resource-name>)  [unwired: 5 in]
                      }
                      frame True {
                      }
                    }
                  }
                  frame True {
                    w1238 = 4 ("Axis")
                    n342 = property on="Property Node" class="DigNum (strict)"(reference=w1233) -> ("Value"=w1234:dbl)  [unwired: 1 in, 2 out]
                    n343 = property on="Property Node" class="DigNum (strict)"(reference=w1235) -> ("Value"=w1237:u32)  [unwired: 1 in, 2 out]
                    n344 = case shown="True" w1243 {
                      tunnel: w1234 -> [w1264 w1266]
                      tunnel: [w1264 w1265] -> w1236
                      frame False {
                      }
                      frame True {
                        n345 = Multiply(x=w1266, y=-1.0) -> (x*y=w1265:dbl)
                      }
                    }
                    n346 = call "Motors Move Constant Velocity.vi"("Axis Multiplier"=w1237, "Axis"=w1238, "error in"=w1241, "VISA in"=w1240, "Speed (mm/s)"=w1236) -> ("error out"=w1242:errorcluster, "VISA out"=w1239:refnum<visa-resource-name>)  [unwired: 5 in]
                    n347 = while {
                      tunnel: w1239 -> [w1254]
                      tunnel: [w1253] -> w1247
                      tunnel: w1242 -> [w1256]
                      tunnel: [w1255] -> w1246
                      tunnel: w1237 -> [w1252]
                      tunnel: w1232 -> [w1251]
                      tunnel: w1231 -> [w1250]
                      tunnel: w1230 -> [w1249]
                      tunnel: w1229 -> [w1248]
                      stop <- w1263 continue-if-true
                      n348 = property on="Property Node" class="Bool (strict)"(reference=w1251) -> ("Value"=w1262:bool)  [unwired: 1 in, 2 out]
                      n349 = property on="Property Node" class="Bool (strict)"(reference=w1250) -> ("Value"=w1261:bool)  [unwired: 1 in, 2 out]
                      n350 = Or(x=w1262, y=w1261) -> (x .or. y?=w1263:bool)
                      n351 = call "Motors Status.vi"("error in"=w1256, "VISA in"=w1254, "Axis"=4, "Axis Multiplier"=w1252) -> ("error out"=w1255:errorcluster, "VISA out"=w1253:refnum<visa-resource-name>, "OS"=w1258:i32, "Actual Position (mm or deg)"=w1259:dbl)  [unwired: 3 in]
                      n352 = property on="Property Node" class="DigNum (strict)"(reference=w1249, "Value"=w1259) -> ()  [unwired: 1 in, 2 out]
                      n353 = call "Motors Decipher Status.vi"("OS"=w1258) -> ("Status"=w1257:string)
                      n354 = property on="Property Node" class="Str"(reference=w1248, "Value"=w1257) -> ()  [unwired: 1 in, 2 out]
                    }
                    n355 = call "Motors Stop.vi"("error in"=w1246, "Axis"=w1238, "VISA in"=w1247) -> ("error out"=w1244:errorcluster, "VISA out"=w1245:refnum<visa-resource-name>)
                  }
                }
              }
              frame #1 {
                n356 = property on="Property Node" class="Bool (strict)"(reference=w1268, "Value"=FALSE) -> ()  [unwired: 1 in, 2 out]
                n357 = property on="Property Node" class="Bool (strict)"(reference=w1269, "Value"=FALSE) -> ()  [unwired: 1 in, 2 out]
              }
            }
          }
        }
        n358 = Unbundle(w176) -> ("X Set Slew Speed?"=w174:refnum<vi>, "(mm/s)"=w168:refnum<vi>, "Y Set Slew Speed?"=w164:refnum<vi>, "(mm/s)"=w167:refnum<vi>, "Z Set Slew Speed?"=w162:refnum<vi>, "(mm/s)"=w166:refnum<vi>, "Theta Set Slew Speed?"=w160:refnum<vi>, "(degrees/s)"=w165:refnum<vi>, "Need to Update Motor Parameters"=w173:refnum<vi>, "X Multiplier"=w172:refnum<vi>, "Y Multiplier"=w171:refnum<vi>, "Z Multiplier"=w170:refnum<vi>, "Theta Multiplier"=w169:refnum<vi>)
        n359 = property on="Property Node" class="Bool (strict)"(reference=w174) -> (reference out=w158:refnum<vi>, "Value"=w175:bool)  [unwired: 1 in, 1 out]
        n360 = case shown="True" w175 {
          tunnel: [w1152 w1160] -> w398
          tunnel: w401 -> [w1152 w1161]
          tunnel: [w1151 w1164] -> w395
          tunnel: w394 -> [w1151 w1165]
          tunnel: w173 -> [_ w1158]
          tunnel: w172 -> [_ w1157]
          tunnel: w168 -> [_ w1156]
          tunnel: w158 -> [_ w1153]
          frame False {
          }
          frame True {
            n361 = property on="Property Node" class="DigNum (strict)"(reference=w1156) -> ("Value"=w1155:dbl)  [unwired: 1 in, 2 out]
            n362 = property on="Property Node" class="DigNum (strict)"(reference=w1157) -> ("Value"=w1159:u32)  [unwired: 1 in, 2 out]
            n363 = property on="Property Node" class="Bool (strict)"(reference=w1153, "Value"=FALSE) -> ()  [unwired: 1 in, 2 out]
            n364 = property on="Property Node" class="Bool (strict)"(reference=w1158, "Value"=TRUE ("Need to Update Motor Parameters")) -> ()  [unwired: 1 in, 2 out]
            n365 = call "Motors Move Speed.vi"("Speed (mm or degree/sec)"=w1155, "error in"=w1165, "VISA in"=w1161, "Axis"=u32 1, "Axis Multiplier"=w1159) -> ("error out"=w1164:errorcluster, "VISA out"=w1160:refnum<visa-resource-name>)  [unwired: 5 in]
          }
        }
        n366 = property on="Property Node" class="Bool (strict)"(reference=w164) -> (reference out=w157:refnum<vi>, "Value"=w163:bool)  [unwired: 1 in, 1 out]
        n367 = case shown="True" w163 {
          tunnel: [w1137 w1146] -> w399
          tunnel: w398 -> [w1137 w1144]
          tunnel: [w1136 w1149] -> w396
          tunnel: w395 -> [w1136 w1150]
          tunnel: w173 -> [_ w1143]
          tunnel: w171 -> [_ w1142]
          tunnel: w167 -> [_ w1141]
          tunnel: w157 -> [_ w1138]
          frame False {
          }
          frame True {
            n368 = property on="Property Node" class="DigNum (strict)"(reference=w1141) -> ("Value"=w1140:dbl)  [unwired: 1 in, 2 out]
            n369 = property on="Property Node" class="DigNum (strict)"(reference=w1142) -> ("Value"=w1145:u32)  [unwired: 1 in, 2 out]
            n370 = property on="Property Node" class="Bool (strict)"(reference=w1138, "Value"=FALSE) -> ()  [unwired: 1 in, 2 out]
            n371 = property on="Property Node" class="Bool (strict)"(reference=w1143, "Value"=TRUE ("Need to Update Motor Parameters")) -> ()  [unwired: 1 in, 2 out]
            n372 = call "Motors Move Speed.vi"("Speed (mm or degree/sec)"=w1140, "error in"=w1150, "VISA in"=w1144, "Axis"=u32 2, "Axis Multiplier"=w1145) -> ("error out"=w1149:errorcluster, "VISA out"=w1146:refnum<visa-resource-name>)  [unwired: 5 in]
          }
        }
        n373 = property on="Property Node" class="Bool (strict)"(reference=w162) -> (reference out=w156:refnum<vi>, "Value"=w161:bool)  [unwired: 1 in, 1 out]
        n374 = case shown="True" w161 {
          tunnel: [w1122 w1131] -> w400
          tunnel: w399 -> [w1122 w1130]
          tunnel: [w1121 w1134] -> w397
          tunnel: w396 -> [w1121 w1135]
          tunnel: w173 -> [_ w1128]
          tunnel: w170 -> [_ w1127]
          tunnel: w166 -> [_ w1126]
          tunnel: w156 -> [_ w1123]
          frame False {
          }
          frame True {
            n375 = property on="Property Node" class="DigNum (strict)"(reference=w1126) -> ("Value"=w1125:dbl)  [unwired: 1 in, 2 out]
            n376 = property on="Property Node" class="DigNum (strict)"(reference=w1127) -> ("Value"=w1129:u32)  [unwired: 1 in, 2 out]
            n377 = property on="Property Node" class="Bool (strict)"(reference=w1123, "Value"=FALSE) -> ()  [unwired: 1 in, 2 out]
            n378 = property on="Property Node" class="Bool (strict)"(reference=w1128, "Value"=TRUE ("Need to Update Motor Parameters")) -> ()  [unwired: 1 in, 2 out]
            n379 = call "Motors Move Speed.vi"("Speed (mm or degree/sec)"=w1125, "error in"=w1135, "VISA in"=w1130, "Axis"=u32 3, "Axis Multiplier"=w1129) -> ("error out"=w1134:errorcluster, "VISA out"=w1131:refnum<visa-resource-name>)  [unwired: 5 in]
          }
        }
        n380 = property on="Property Node" class="Bool (strict)"(reference=w160) -> (reference out=w155:refnum<vi>, "Value"=w159:bool)  [unwired: 1 in, 1 out]
        n381 = case shown="True" w159 {
          tunnel: [w1107 w1116] -> w392
          tunnel: w400 -> [w1107 w1115]
          tunnel: [w1106 w1117] -> w393
          tunnel: w397 -> [w1106 w1120]
          tunnel: w173 -> [_ w1113]
          tunnel: w169 -> [_ w1112]
          tunnel: w165 -> [_ w1111]
          tunnel: w155 -> [_ w1108]
          frame False {
          }
          frame True {
            n382 = property on="Property Node" class="DigNum (strict)"(reference=w1111) -> ("Value"=w1110:dbl)  [unwired: 1 in, 2 out]
            n383 = property on="Property Node" class="DigNum (strict)"(reference=w1112) -> ("Value"=w1114:u32)  [unwired: 1 in, 2 out]
            n384 = property on="Property Node" class="Bool (strict)"(reference=w1113, "Value"=TRUE ("Need to Update Motor Parameters")) -> ()  [unwired: 1 in, 2 out]
            n385 = property on="Property Node" class="Bool (strict)"(reference=w1108, "Value"=FALSE) -> ()  [unwired: 1 in, 2 out]
            n386 = call "Motors Move Speed.vi"("Speed (mm or degree/sec)"=w1110, "error in"=w1120, "VISA in"=w1115, "Axis"=u32 4, "Axis Multiplier"=w1114) -> ("error out"=w1117:errorcluster, "VISA out"=w1116:refnum<visa-resource-name>)  [unwired: 5 in]
          }
        }
        n387 = Unbundle(w154) -> ("Status X"=w153:refnum<vi>, "X-Axis (mm)"=w152:refnum<vi>, "X Multiplier"=w151:refnum<vi>, "X Moving"=w150:refnum<vi>, "Status Y"=w149:refnum<vi>, "Y-Axis (mm)"=w148:refnum<vi>, "Y Multiplier"=w147:refnum<vi>, "Y Moving"=w146:refnum<vi>, "Status Z"=w145:refnum<vi>, "Z-Axis (mm)"=w144:refnum<vi>, "Z Multiplier"=w143:refnum<vi>, "Z Moving"=w142:refnum<vi>, "Status Theta"=w141:refnum<vi>, "Theta (deg)"=w140:refnum<vi>, "Theta Multiplier"=w139:refnum<vi>, "Theta Moving"=w138:refnum<vi>)
        n388 = Quotient & Remainder(x=w369, y=4) -> (x-y*floor(x/y)=w390:i32)  [unwired: 1 out]
        n389 = case shown="0, Default" w390 {
          tunnel: w393 -> [w982 w1000 w1017 w1036]
          tunnel: w392 -> [w983 w1001 w1019 w1037]
          tunnel: [w981 w998 w1016 w1035] -> w388
          tunnel: [w980 w999 w1018 w1034] -> w387
          tunnel: w153 -> [w978 _ _ _]
          tunnel: w152 -> [w977 _ _ _]
          tunnel: w151 -> [w976 _ _ _]
          tunnel: w150 -> [w975 _ _ _]
          tunnel: w149 -> [_ w996 _ _]
          tunnel: w148 -> [_ w995 _ _]
          tunnel: w147 -> [_ w994 _ _]
          tunnel: w146 -> [_ w993 _ _]
          tunnel: w145 -> [_ _ w1014 _]
          tunnel: w144 -> [_ _ w1013 _]
          tunnel: w143 -> [_ _ w1012 _]
          tunnel: w142 -> [_ _ w1011 _]
          tunnel: w141 -> [_ _ _ w1032]
          tunnel: w140 -> [_ _ _ w1031]
          tunnel: w139 -> [_ _ _ w1030]
          tunnel: w138 -> [_ _ _ w1029]
          frame 0, Default {
            n390 = property on="Property Node" class="DigNum (strict)"(reference=w976) -> ("Value"=w979:u32)  [unwired: 1 in, 2 out]
            n391 = call "Motors Status.vi"("error in"=w982, "VISA in"=w983, "Axis"=1, "Axis Multiplier"=w979) -> ("error out"=w981:errorcluster, "VISA out"=w980:refnum<visa-resource-name>, "OS"=w989:i32, "Actual Position (mm or deg)"=w984:dbl)  [unwired: 3 in]
            n392 = property on="Property Node" class="DigNum (strict)"(reference=w977, "Value"=w984) -> ()  [unwired: 1 in, 2 out]
            n393 = call "Motors Decipher Status.vi"("OS"=w989) -> ("Status"=w988:string)
            n394 = property on="Property Node" class="Str"(reference=w978, "Value"=w988) -> ()  [unwired: 1 in, 2 out]
            n395 = Equal?(x=w988, y="Idle") -> (x = y?=w986:bool)
            n396 = case shown="False" w986 {
              tunnel: [TRUE FALSE] -> w985
              frame False {
              }
              frame True {
              }
            }
            n397 = property on="Property Node" class="Bool (strict)"(reference=w975, "Value"=w985) -> ()  [unwired: 1 in, 2 out]
          }
          frame 1 {
            n398 = property on="Property Node" class="DigNum (strict)"(reference=w994) -> ("Value"=w997:u32)  [unwired: 1 in, 2 out]
            n399 = call "Motors Status.vi"("error in"=w1000, "VISA in"=w1001, "Axis"=2, "Axis Multiplier"=w997) -> ("error out"=w998:errorcluster, "VISA out"=w999:refnum<visa-resource-name>, "OS"=w1006:i32, "Actual Position (mm or deg)"=w1007:dbl)  [unwired: 3 in]
            n400 = property on="Property Node" class="DigNum (strict)"(reference=w995, "Value"=w1007) -> ()  [unwired: 1 in, 2 out]
            n401 = call "Motors Decipher Status.vi"("OS"=w1006) -> ("Status"=w1004:string)
            n402 = property on="Property Node" class="Str"(reference=w996, "Value"=w1004) -> ()  [unwired: 1 in, 2 out]
            n403 = Equal?(x=w1004, y="Idle") -> (x = y?=w1003:bool)
            n404 = case shown="False" w1003 {
              tunnel: [TRUE FALSE] -> w1002
              frame False {
              }
              frame True {
              }
            }
            n405 = property on="Property Node" class="Bool (strict)"(reference=w993, "Value"=w1002) -> ()  [unwired: 1 in, 2 out]
          }
          frame 2 {
            n406 = property on="Property Node" class="DigNum (strict)"(reference=w1012) -> ("Value"=w1015:u32)  [unwired: 1 in, 2 out]
            n407 = call "Motors Status.vi"("error in"=w1017, "VISA in"=w1019, "Axis"=3, "Axis Multiplier"=w1015) -> ("error out"=w1016:errorcluster, "VISA out"=w1018:refnum<visa-resource-name>, "OS"=w1024:i32, "Actual Position (mm or deg)"=w1025:dbl)  [unwired: 3 in]
            n408 = property on="Property Node" class="DigNum (strict)"(reference=w1013, "Value"=w1025) -> ()  [unwired: 1 in, 2 out]
            n409 = call "Motors Decipher Status.vi"("OS"=w1024) -> ("Status"=w1022:string)
            n410 = property on="Property Node" class="Str"(reference=w1014, "Value"=w1022) -> ()  [unwired: 1 in, 2 out]
            n411 = Equal?(x=w1022, y="Idle") -> (x = y?=w1021:bool)
            n412 = case shown="False" w1021 {
              tunnel: [TRUE FALSE] -> w1020
              frame False {
              }
              frame True {
              }
            }
            n413 = property on="Property Node" class="Bool (strict)"(reference=w1011, "Value"=w1020) -> ()  [unwired: 1 in, 2 out]
          }
          frame 3 {
            n414 = property on="Property Node" class="DigNum (strict)"(reference=w1030) -> ("Value"=w1033:u32)  [unwired: 1 in, 2 out]
            n415 = call "Motors Status.vi"("error in"=w1036, "VISA in"=w1037, "Axis"=4, "Axis Multiplier"=w1033) -> ("error out"=w1035:errorcluster, "VISA out"=w1034:refnum<visa-resource-name>, "OS"=w1042:i32, "Actual Position (mm or deg)"=w1043:dbl)  [unwired: 3 in]
            n416 = property on="Property Node" class="DigNum (strict)"(reference=w1031, "Value"=w1043) -> ()  [unwired: 1 in, 2 out]
            n417 = call "Motors Decipher Status.vi"("OS"=w1042) -> ("Status"=w1040:string)
            n418 = property on="Property Node" class="Str"(reference=w1032, "Value"=w1040) -> ()  [unwired: 1 in, 2 out]
            n419 = Equal?(x=w1040, y="Idle") -> (x = y?=w1039:bool)
            n420 = case shown="True" w1039 {
              tunnel: [TRUE FALSE] -> w1038
              frame False {
              }
              frame True {
              }
            }
            n421 = property on="Property Node" class="Bool (strict)"(reference=w1029, "Value"=w1038) -> ()  [unwired: 1 in, 2 out]
          }
        }
        n422 = Unbundle(w137) -> ("Go To Saved Position?"=w135:refnum<vi>, "Defined Positions"=w133:refnum<vi>)  [unwired: 5 out]
        n423 = property on="Property Node" class="Bool (strict)"(reference=w135) -> (reference out=w134:refnum<vi>, "Value"=w136:bool)  [unwired: 1 in, 1 out]
        n424 = case shown="True" w136 {
          tunnel: w388 -> [w941 w947]
          tunnel: w387 -> [w940 w953]
          tunnel: [w941 w966] -> w386
          tunnel: [w940 w965] -> w385
          tunnel: w134 -> [_ w944]
          tunnel: w133 -> [_ w943]
          frame False {
          }
          frame True {
            w963 = 4 ("index (row)")
            w961 = 3 ("index (row)")
            w958 = 2 ("index (row)")
            w955 = 1 ("index (row)")
            n425 = property on="Property Node" class="LstBox (strict)"(reference=w943) -> ("Value"=w942:i32)  [unwired: 1 in, 2 out]
            n426 = property on="Property Node" class="Path"() -> ("Value"=w948:path)  [unwired: 2 in, 2 out]
            n427 = call "Motors Position Load.vi"("error in"=w947, "file path"=w948) -> ("error out"=w946:errorcluster, "Positions"=w969:string[][])
            n428 = property on="Property Node" class="Bool (strict)"(reference=w944, "Value"=FALSE) -> ()  [unwired: 1 in, 2 out]
            n429 = property on="Property Node" class="DigNum (strict)"() -> ("Value"=w952:u32)  [unwired: 2 in, 2 out]
            n430 = Index Array(array=w969, index (row)=w963, index (col)=w942) -> (element=w970:string)
            n431 = Index Array(array=w969, index (row)=w961, index (col)=w942) -> (element=w971:string)
            n432 = Index Array(array=w969, index (row)=w958, index (col)=w942) -> (element=w973:string)
            n433 = Index Array(array=w969, index (row)=w955, index (col)=w942) -> (element=w974:string)
            n434 = Fract/Exp String To Number(string=w970) -> (number=w964:dbl)  [unwired: 3 in, 1 out]
            n435 = Fract/Exp String To Number(string=w971) -> (number=w960:dbl)  [unwired: 3 in, 1 out]
            n436 = Fract/Exp String To Number(string=w973) -> (number=w957:dbl)  [unwired: 3 in, 1 out]
            n437 = Fract/Exp String To Number(string=w974) -> (number=w954:dbl)  [unwired: 3 in, 1 out]
            n438 = property on="Property Node" class="DigNum (strict)"() -> ("Value"=w951:u32)  [unwired: 2 in, 2 out]
            n439 = property on="Property Node" class="DigNum (strict)"() -> ("Value"=w950:u32)  [unwired: 2 in, 2 out]
            n440 = call "Motors Move Absolute.vi"("Axis Multiplier"=w952, "Axis"=w955, "error in"=w946, "VISA in"=w953, "Position (mm or degree)"=w954) -> ("error out"=w972:errorcluster, "VISA out"=w956:refnum<visa-resource-name>)  [unwired: 5 in]
            n441 = property on="Property Node" class="DigNum (strict)"() -> ("Value"=w949:u32)  [unwired: 2 in, 2 out]
            n442 = call "Motors Move Absolute.vi"("Axis Multiplier"=w951, "Axis"=w958, "error in"=w972, "VISA in"=w956, "Position (mm or degree)"=w957) -> ("error out"=w968:errorcluster, "VISA out"=w959:refnum<visa-resource-name>)  [unwired: 5 in]
            n443 = call "Motors Move Absolute.vi"("Axis Multiplier"=w950, "Axis"=w961, "error in"=w968, "VISA in"=w959, "Position (mm or degree)"=w960) -> ("error out"=w967:errorcluster, "VISA out"=w962:refnum<visa-resource-name>)  [unwired: 5 in]
            n444 = call "Motors Move Absolute.vi"("Axis Multiplier"=w949, "Axis"=w963, "error in"=w967, "VISA in"=w962, "Position (mm or degree)"=w964) -> ("error out"=w966:errorcluster, "VISA out"=w965:refnum<visa-resource-name>)  [unwired: 5 in]
          }
        }
        n445 = property on="Property Node" class="Bool (strict)"() -> ("Value"=w391:bool)  [unwired: 2 in, 2 out]
        n446 = case shown="True" w391 {
          tunnel: w386 -> [w1048 w1051]
          tunnel: w385 -> [w1047 w1052]
          tunnel: [w1047 w1050] -> _
          tunnel: [w1048 w1049] -> w376
          frame False {
          }
          frame True {
            n447 = property on="Property Node" class="Bool (strict)"("Value"=FALSE ("Need to Update Motor Parameters")) -> ()  [unwired: 2 in, 2 out]
            n448 = flat-sequence {
              tunnel: w1052 -> [w1058]
              tunnel: w1051 -> [w1057]
              tunnel: [w1056] -> w1050
              tunnel: [w1055] -> w1049
              frame #0 {
                n449 = call <vilib>:"Set Busy.vi"() -> ()  [unwired: 10 in, 2 out]
                n450 = property on="Property Node" class="Str"("Value"="Updating Motor Parameters\nThis Should Take About 5 Seconds" ("Status Theta")) -> ()  [unwired: 2 in, 2 out]
              }
              frame #1 {
                n451 = call "Motors Status Verbose.vi"("Axis"=1, "VISA in"=w1058, "error in"=w1057) -> ("Slew Speed (mm or deg/s)"=w1074:dbl, "Jogger Normal Speed (mm or deg/s)"=w1075:dbl, "Jogger Fast Speed (mm or deg/s)"=w1076:dbl, "Actual Position (mm or deg)"=w1091:dbl, "OS"=w1065:i32, "Mode"=w1100:string, "VISA out"=w1080:refnum<visa-resource-name>, "error out"=w1062:errorcluster)  [unwired: 4 in, 1 out]
                n452 = property on="Property Node" class="Str"("Value"=w1100) -> ()  [unwired: 2 in, 2 out]
                n453 = property on="Property Node" class="DigNum (strict)"("Value"=w1074) -> ()  [unwired: 2 in, 2 out]
                n454 = property on="Property Node" class="DigNum (strict)"("Value"=w1075) -> ()  [unwired: 2 in, 2 out]
                n455 = property on="Property Node" class="DigNum (strict)"("Value"=w1076) -> ()  [unwired: 2 in, 2 out]
                n456 = property on="Property Node" class="DigNum (strict)"("Value"=w1091) -> ()  [unwired: 2 in, 2 out]
                n457 = call "Motors Decipher Status.vi"("OS"=w1065) -> ("Status"=w1102:string)
                n458 = call "Motors Status Verbose.vi"("Axis"=2, "VISA in"=w1080, "error in"=w1062) -> ("Slew Speed (mm or deg/s)"=w1077:dbl, "Jogger Normal Speed (mm or deg/s)"=w1078:dbl, "Jogger Fast Speed (mm or deg/s)"=w1079:dbl, "Actual Position (mm or deg)"=w1092:dbl, "OS"=w1066:i32, "Mode"=w1101:string, "VISA out"=w1081:refnum<visa-resource-name>, "error out"=w1063:errorcluster)  [unwired: 4 in, 1 out]
                n459 = property on="Property Node" class="Str"("Value"=w1102) -> ()  [unwired: 2 in, 2 out]
                n460 = property on="Property Node" class="Str"("Value"=w1101) -> ()  [unwired: 2 in, 2 out]
                n461 = property on="Property Node" class="DigNum (strict)"("Value"=w1077) -> ()  [unwired: 2 in, 2 out]
                n462 = property on="Property Node" class="DigNum (strict)"("Value"=w1078) -> ()  [unwired: 2 in, 2 out]
                n463 = property on="Property Node" class="DigNum (strict)"("Value"=w1079) -> ()  [unwired: 2 in, 2 out]
                n464 = property on="Property Node" class="DigNum (strict)"("Value"=w1092) -> ()  [unwired: 2 in, 2 out]
                n465 = call "Motors Decipher Status.vi"("OS"=w1066) -> ("Status"=w1093:string)
                n466 = call "Motors Status Verbose.vi"("Axis"=3, "VISA in"=w1081, "error in"=w1063) -> ("Slew Speed (mm or deg/s)"=w1090:dbl, "Jogger Normal Speed (mm or deg/s)"=w1089:dbl, "Jogger Fast Speed (mm or deg/s)"=w1088:dbl, "Actual Position (mm or deg)"=w1087:dbl, "OS"=w1067:i32, "Mode"=w1094:string, "VISA out"=w1082:refnum<visa-resource-name>, "error out"=w1064:errorcluster)  [unwired: 4 in, 1 out]
                n467 = Not Equal?(x=w1102, y="Idle") -> (x != y?=w1083:bool)
                n468 = property on="Property Node" class="Str"("Value"=w1093) -> ()  [unwired: 2 in, 2 out]
                n469 = property on="Property Node" class="Str"("Value"=w1094) -> ()  [unwired: 2 in, 2 out]
                n470 = property on="Property Node" class="DigNum (strict)"("Value"=w1090) -> ()  [unwired: 2 in, 2 out]
                n471 = property on="Property Node" class="DigNum (strict)"("Value"=w1089) -> ()  [unwired: 2 in, 2 out]
                n472 = property on="Property Node" class="DigNum (strict)"("Value"=w1088) -> ()  [unwired: 2 in, 2 out]
                n473 = property on="Property Node" class="DigNum (strict)"("Value"=w1087) -> ()  [unwired: 2 in, 2 out]
                n474 = property on="Property Node" class="Bool (strict)"("Value"=w1083) -> ()  [unwired: 2 in, 2 out]
                n475 = call "Motors Status Verbose.vi"("Axis"=4, "VISA in"=w1082, "error in"=w1064) -> ("Slew Speed (mm or deg/s)"=w1096:dbl, "Jogger Normal Speed (mm or deg/s)"=w1097:dbl, "Jogger Fast Speed (mm or deg/s)"=w1098:dbl, "Actual Position (mm or deg)"=w1099:dbl, "OS"=w1068:i32, "Mode"=w1103:string, "VISA out"=w1056:refnum<visa-resource-name>, "error out"=w1055:errorcluster)  [unwired: 4 in, 1 out]
                n476 = call "Motors Decipher Status.vi"("OS"=w1067) -> ("Status"=w1095:string)
                n477 = Not Equal?(x=w1093, y="Idle") -> (x != y?=w1084:bool)
                n478 = property on="Property Node" class="DigNum (strict)"("Value"=w1096) -> ()  [unwired: 2 in, 2 out]
                n479 = property on="Property Node" class="DigNum (strict)"("Value"=w1097) -> ()  [unwired: 2 in, 2 out]
                n480 = property on="Property Node" class="DigNum (strict)"("Value"=w1098) -> ()  [unwired: 2 in, 2 out]
                n481 = property on="Property Node" class="DigNum (strict)"("Value"=w1099) -> ()  [unwired: 2 in, 2 out]
                n482 = property on="Property Node" class="Str"("Value"=w1095) -> ()  [unwired: 2 in, 2 out]
                n483 = property on="Property Node" class="Str"("Value"=w1103) -> ()  [unwired: 2 in, 2 out]
                n484 = call "Motors Decipher Status.vi"("OS"=w1068) -> ("Status"=w1104:string)
                n485 = property on="Property Node" class="Bool (strict)"("Value"=w1084) -> ()  [unwired: 2 in, 2 out]
                n486 = property on="Property Node" class="Str"("Value"=w1104) -> ()  [unwired: 2 in, 2 out]
                n487 = Not Equal?(x=w1095, y="Idle") -> (x != y?=w1085:bool)
                n488 = Not Equal?(x=w1104, y="Idle") -> (x != y?=w1086:bool)
                n489 = property on="Property Node" class="Bool (strict)"("Value"=w1085) -> ()  [unwired: 2 in, 2 out]
                n490 = property on="Property Node" class="Bool (strict)"("Value"=w1086) -> ()  [unwired: 2 in, 2 out]
              }
              frame #2 {
                n491 = call <vilib>:"Unset Busy.vi"() -> ()  [unwired: 11 in, 1 out]
                n492 = property on="Property Node" class="Str"("Value"="Running" ("Status Theta")) -> ()  [unwired: 2 in, 2 out]
              }
            }
          }
        }
        n493 = property on="Property Node" class="Clust (strict)"("Value"=w376) -> ()  [unwired: 2 in, 2 out]
        "Loop i" <- w369
      }
    }
  }
  n494 = property on="Property Node" class="Bool (strict)"(reference=w73, "Value"=w107) -> ()  [unwired: 1 in, 2 out]
